vi "Dashboard Main.vi"() -> ()   [LabVIEW 2017]
uses:
  <vilib>/Utility/miscctls.llb/LVRowAndColumnTypeDef.ctl
  <vilib>/event_ctls.llb/eventvkey.ctl
  <vilib>/Rock Robotics/Network Tables/NT Read Numeric Array.vi
  <vilib>/Rock Robotics/Network Tables/NT Write Boolean.vi
  <vilib>/Rock Robotics/WPI/Dashboard/WPI_DashboardLogging Global.vi
panel:
  in  "Camera Settings Right":T1={"Frame Rate"=30, "Compression"=30, "Size"=1, "DB Camera Config"=FALSE} {"Frame Rate" scale=1.0..30.0; "Compression" scale=100.0..-1.0; "Size" items=["640x480", "320x240", "160x120"]}
  in  "Camera Name Right":string(combo)="No Camera Selection"
  out "Camera Info":cluster{"Mbps LED":bool, "Mbps":dbl, "fps":dbl} {"fps" format="%#.1g"; "Mbps" format="%#.1g"}
  in  "Camera Settings":T1={"Frame Rate"=30, "Compression"=30, "Size"=1, "DB Camera Config"=FALSE} {"Frame Rate" scale=1.0..30.0; "Compression" scale=100.0..-1.0; "Size" items=["640x480", "320x240", "160x120"]}
  in  "TCP":refnum<k5>
  in  "Rec Mode":enum32{"Stop", "Record", "Playback"}(radio)
  out "Robot IP":string
  out "Image Message":string="Timeout in Camera Communications"
  in  "Dashboard Tab":T2(tab)
  in  "Select Auto":string(combo)="Select Autonomous ..."
  out "NT Connection":bool
  out "MotorChart R":cluster{"Numeric":dbl, "Numeric":dbl}(graph)
  out "MotorChart L":cluster{"Numeric":dbl, "Numeric":dbl}(graph)
  out "MotorSliders R":cluster{"MotorSlide1":dbl, "MotorSlide2":dbl} {"MotorSlide2" scale=-1.0..1.0 scale format="%#_2e"; "MotorSlide1" scale=-1.0..1.0 scale format="%#_2e"}
  out "MotorSliders L":cluster{"MotorSlide1":dbl, "MotorSlide2":dbl} {"MotorSlide2" scale=-1.0..1.0 scale format="%#_2e"; "MotorSlide1" scale=-1.0..1.0 scale format="%#_2e"}
  out "Gyro":dbl(knob) scale=0.0..360.0
  out "JS1 Z":dbl(slide) scale=-1.0..1.0 scale format="%#_2e"
  out "JS1 Graph":cluster{"X":dbl, "Y":dbl}[](graph)
  out "JS1 Buttons":T3
  out "JS2 Z":dbl(slide) scale=-1.0..1.0 scale format="%#_2e"
  out "JS2 Graph":cluster{"X":dbl, "Y":dbl}[](graph)
  out "JS2 Buttons":T3
  out "Mode":T4(ring)=enum."Auto Disabled"
  out "Camera Image Right":T5(plugin-control)
  in  "DB/String 9":string
  in  "DB/String 8":string
  in  "DB/String 7":string
  in  "DB/String 6":string
  in  "DB/String 5":string
  in  "DB/String 4":string
  in  "DB/String 3":string
  in  "DB/String 2":string
  in  "DB/String 1":string
  in  "DB/String 0":string
  in  "DB/Slider 0":dbl(slide) scale=0.0..5.0
  in  "DB/Slider 1":dbl(slide) scale=0.0..5.0
  in  "DB/Slider 2":dbl(slide) scale=0.0..5.0
  in  "DB/Slider 3":dbl(slide) scale=0.0..5.0
  out "DB/LED 3":bool
  out "DB/LED 2":bool
  out "DB/LED 1":bool
  out "DB/LED 0":bool
  in  "DB/Button 3":bool
  in  "DB/Button 2":bool
  in  "DB/Button 1":bool
  in  "DB/Button 0":bool caption="New Name"
  out "Elev Encoder":dbl
  out "Fused Heading":dbl
  out "Right Encoder":dbl
  out "Left Encoder":dbl
  in  "Cross Line":bool
  in  "Do Nothing":bool
  in  "Cross? Button":bool
  in  "Three Cube Button":bool
  in  "Two Cube Button":bool
  in  "One Cube Button":bool
  in  "Switch Button":bool
  in  "Scale Button":bool
  in  "Right Button":bool
  in  "Center Button":bool
  in  "Left Button":bool
  out "Game Data":string
  out "AutonControl":string
  out "Reboot?":bool caption="Boolean"
  in  "Test Slider":dbl(slide) scale=0.0..100.0 scale format="%#_3g"
  in  "On/Off":bool caption="Solenoid"
  in  "Test Name":u16(ring) items=["Select the test to run..."]
  in  "Test Tree":string(tree)
  in  "Motor":cluster{"Value":dbl, "Enable":bool} {"Value" scale=-1.0..1.0 scale format="%#_3g"}
  out "Progress":T6 {"Test Progress" scale=0.0..100.0}
  in  "Rev/Fwd":cluster{"Forward":bool, "Reverse":bool}
  in  "Test Ring":u16(ring) items=["Monochrome", "Color"]
  out "Cmd Status":string
  in  "Execute Command":bool
  in  "Command Params":string[][](table)
  in  "Command Selection":i32(listbox)
  in  "CheckList":i32(listbox)
  out "Tree":string(tree)
  out "Camera Image":T5(plugin-control)
  out "Background":bool
  in  "Camera Name":string(combo)="No Camera Selection"
  # "HW"
  # "HW"
  # "Joysticks"
  # "Drive Motors"
  # "Front"
  # "Right"
  # "Left"
  # "Back"
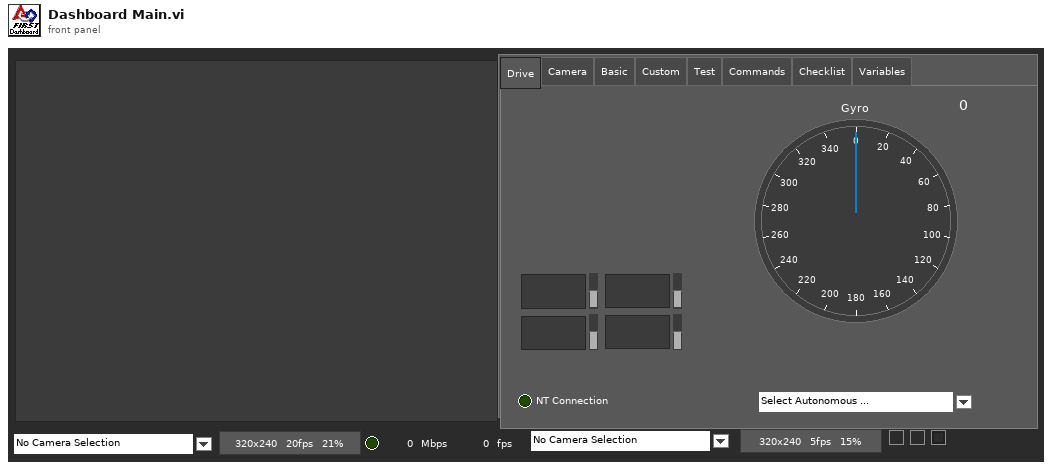
[diagram p1: front panel]
types:
  T1 = cluster{"Frame Rate":i32, "Compression":i32, "Size":u16, "DB Camera Config":bool}
  T2 = enum32{"Drive", "Camera", "Basic", "Custom", "Test", "Commands", "Checklist", "Variables"}
  T3 = cluster{bool, bool, bool, bool, bool, bool, bool, bool, bool, bool, bool, bool}
  T4 = enum8{"Tele-Op Disabled", "Tele-Op Enabled", "Auto Disabled", "Auto Enabled", "Test Disabled", "Test Enabled", "Disconnected", "No Code", "E-Stop"}
  T5 = typedef "IMAQ Image.ctl" = refnum<image>
  T6 = cluster{"Test Progress":u8, "Test Progress Text":string}
  T7 = cluster{"Save Path":path, "Interval (s)":dbl, "Keep":i32}
  T8 = typedef "Image Type" = u32
  T9 = cluster{"IDs":cluster{"RPC field ID":u16, "Unique ID":u16}, "String":string}
  T10 = cluster{"Error Strings":string, "Disable Counts":cluster{u16, u16}, "Rail Faults":cluster{u16, u16, u16}, "Robot IP":string, "DB Mode":u8, "Event Info":cluster{"Name":string, "Type":u8, "Number":u16, "Replay":u8}}
  T11 = cluster{"Storage":cluster{"Disk Free":u64, "RAM Block":u32, "RAM free":u32}, "CPU Utilization":cluster{"CPU % ISR":sgl, "CPU % Time Crit":sgl, "CPU % Timed Str":sgl, "CPU % High":sgl, "CPU % Above":sgl, "CPU % Normal":sgl, "CPU % Low":sgl}, "CAN":cluster{"% Bus Utilization":sgl, "Bus Off Cnt":u32, "TX_FIFO Full Cnt":u32, "Receive Error Cnt":u8, "Transmit Error Cnt":u8}, "HID":cluster{"HID Outputs":u32, "Rumble Low":u16, "Rumble High":u16}[]}
  T12 = cluster{"Status bits":cluster{"Test Mode":bool, "Autonomous":bool, "Enabled":bool, "Code Start":bool, "Brownout":bool, "Reserved 2":bool, "Reserved 3":bool, "E-Stop":bool}, "Code Trace":cluster{"Disabled":bool, "TeleOp":bool, "Auto":bool, "Test":bool}, "Controller Type":enum16{"unknown", "cRIO", "roboRio"}, "Code?":enum16{"unknown", "noCode", "code"}, "Battery V":dbl}
  T13 = cluster{"Control Bits":cluster{"TestMode":bool, "Autonomous":bool, "Enabled":bool, "FMS Present":bool, bool, bool, bool, "E-Stop":bool}, "Team Station ":u8, "Countdown":sgl, "Joystick Values":cluster{"Axes":dbl[], "Buttons":bool[], "POVs":i16[]}[]}
  T14 = cluster{"Axes":dbl[], "Buttons":bool[], "POVs":i16[]}[]
  T15 = cluster{"Axes":dbl[], "Buttons":bool[], "POVs":i16[]}
  T16 = cluster{"Buttons[0]":bool, "Buttons[1]":bool, "Buttons[2]":bool, "Buttons[3]":bool, "Buttons[4]":bool, "Buttons[5]":bool, "Buttons[6]":bool, "Buttons[7]":bool, "Buttons[8]":bool, "Buttons[9]":bool, "Buttons[10]":bool, "Buttons[11]":bool}
  T17 = cluster{"Camera Image":refnum<vi>, "Dashboard Tab":refnum<vi>, "Background":refnum<vi>, "Rec Mode":refnum<vi>, "Test Slider":refnum<vi>, "On/Off ":refnum<vi>, "Test Ring":refnum<vi>, "Rev/Fwd":refnum<vi>, "Test Name":refnum<vi>, "Motor":refnum<vi>, "Progress":refnum<vi>, "CheckList":refnum<vi>, "Tree":refnum<vi>, "Test Tree":refnum<vi>, "Command Params":refnum<vi>, "Command Selection":refnum<vi>, "Execute Command":refnum<vi>, "Cmd Status":refnum<vi>, "Camera Settings":refnum<vi>, "Camera Name":refnum<vi>, "Camera Info":refnum<vi>, "Camera Settings Right":refnum<vi>, "Camera Name Right":refnum<vi>, "Camera Image Right":refnum<vi>}
  T18 = cluster{"Camera Name":string, string, "Saved DB Images Info":cluster{"Save Path":path, "Interval (s)":dbl, "Keep":i32}}
  T19 = cluster{"Camera Name Right":string, string, "Saved DB Images Info":cluster{"Save Path":path, "Interval (s)":dbl, "Keep":i32}}
  T20 = cluster{"Operation":enum16{"Update", "Clear"}, "Color Box":u32}[]
  T21 = typedef "eventvkey.ctl" = enum16{"ASCII", "Enter", "Return", "Shift", "Ctrl", "Alt", "Cmd", "Opt", "Caps", "NumLock", "Clear", "Break", "Up", "Down", "Left", "Right", "Insert", "Delete", "Home", "End", "PageUp", "PageDown", "Escape", "Help", "Pause", "ScrollLock", "F1", "F2", "F3", "F4", "F5", "F6", "F7", "F8", "F9", "F10", "F11", "F12", "F13", "F14", "F15", "F16", "F17", "F18", "F19", "F20", "F21", "F22", "F23", "F24", "Play", "VolumeUp", "VolumeDown", "Mute", "Two Byte Char"}
  T22 = cluster{"Image Size":bool, "Image Type":bool, "Pixel Value":bool, "ROI Information":bool, "Zoom Factor":bool}
  T23 = cluster{"Operation":enum16{"Update", "Clear"}, "Color Box":u32}
  T24 = typedef "LVRowAndColumnTypeDef.ctl" = cluster{"Row":i32, "Column":i32}
  T25 = cluster{"Shift":bool, "Ctrl":bool, "Alt":bool, "Cmd":bool, "Opt":bool}
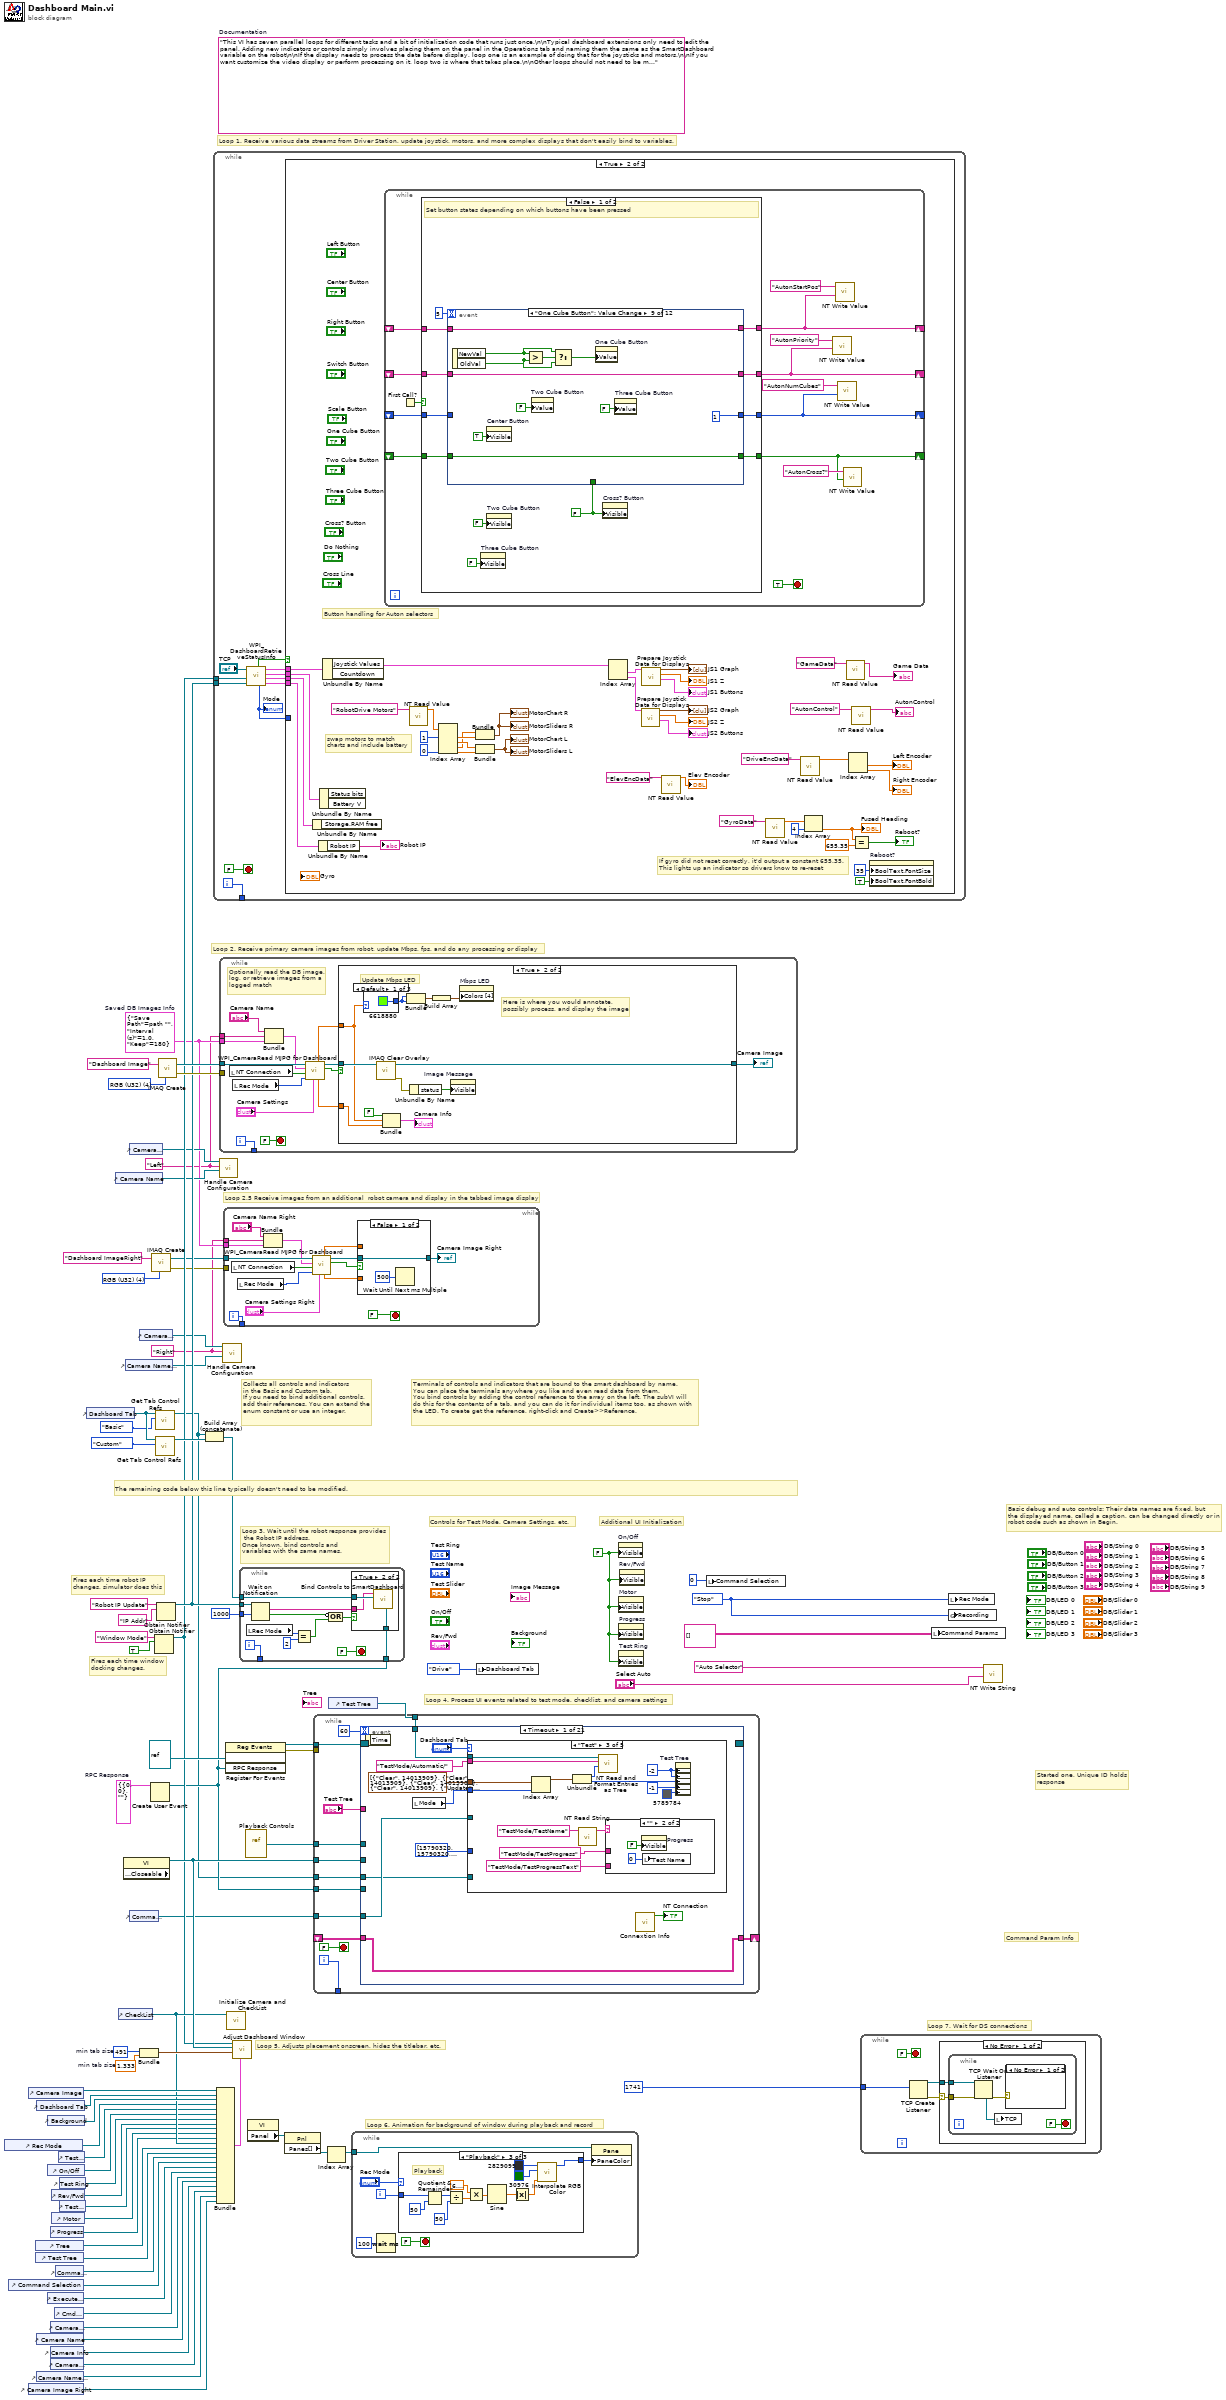
[diagram p0: block diagram]
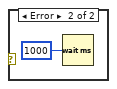
[diagram p3: hidden frame]
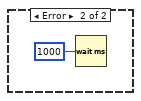
[diagram p4: hidden frame]
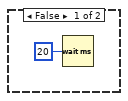
[diagram p5: hidden frame]
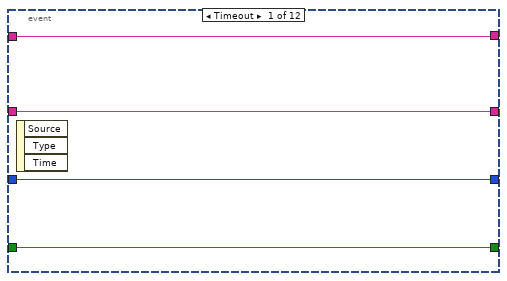
[diagram p6: hidden frame]
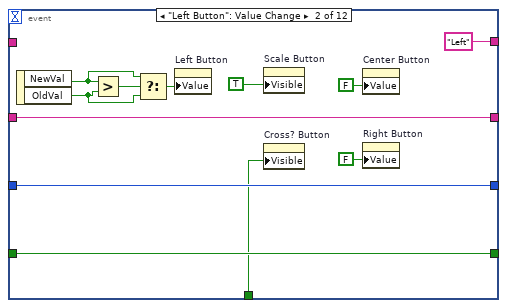
[diagram p7: hidden frame]
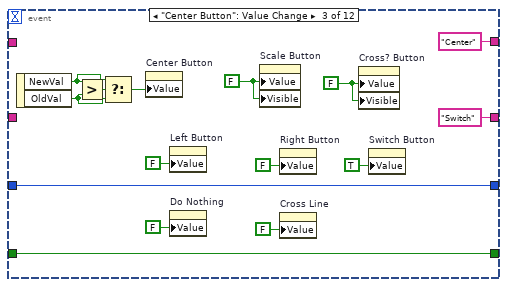
[diagram p8: hidden frame]
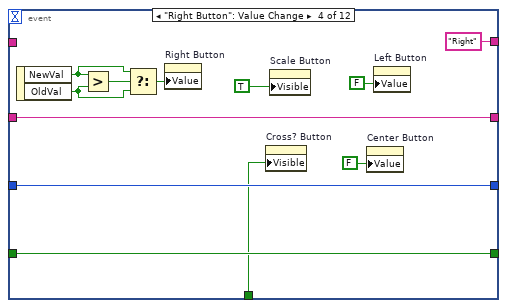
[diagram p9: hidden frame]
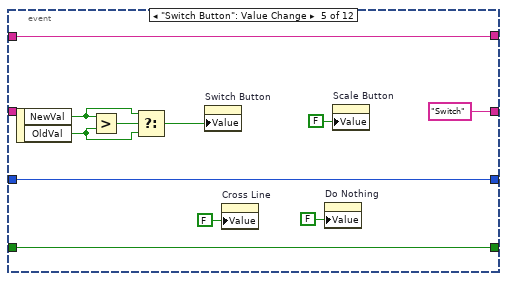
[diagram p10: hidden frame]
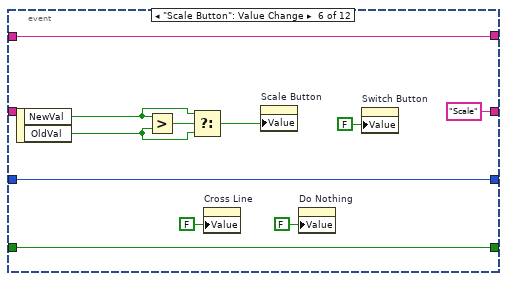
[diagram p11: hidden frame]
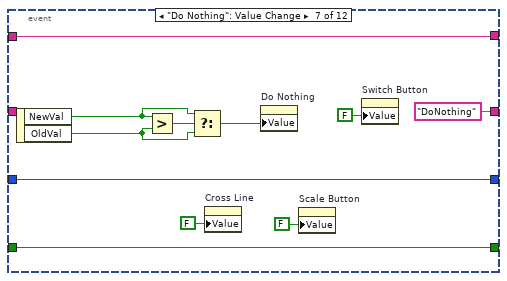
[diagram p12: hidden frame]
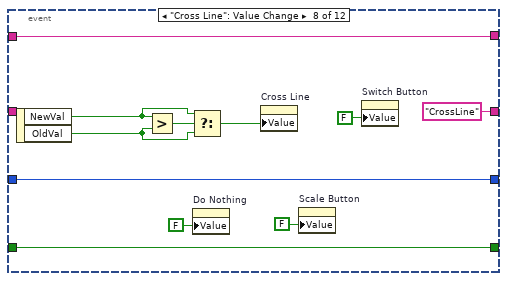
[diagram p13: hidden frame]
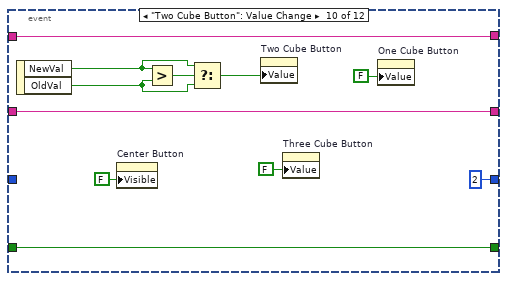
[diagram p14: hidden frame]
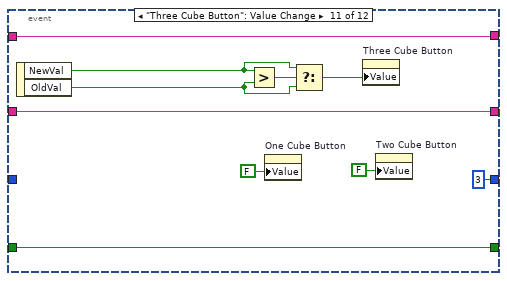
[diagram p15: hidden frame]
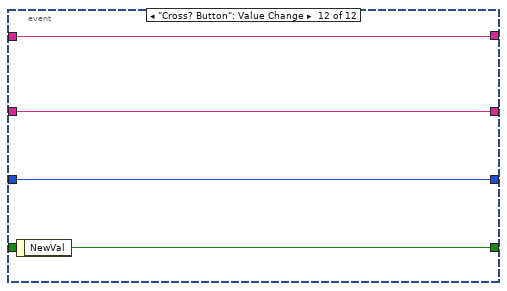
[diagram p16: hidden frame]
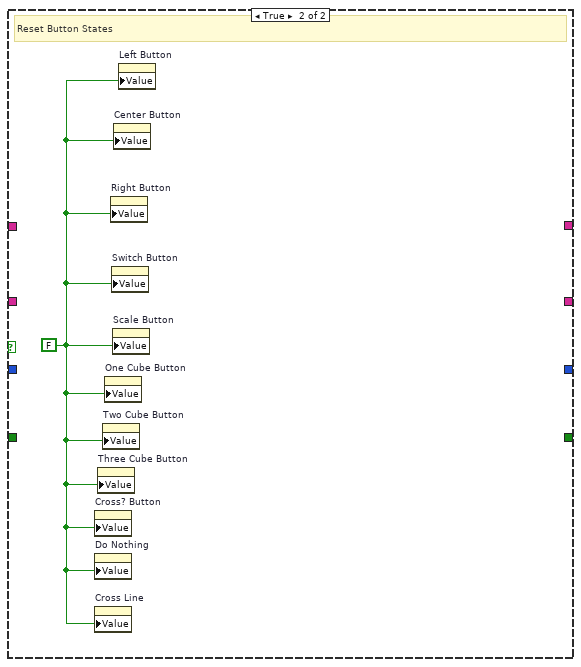
[diagram p17: hidden frame]
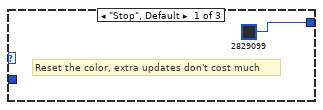
[diagram p18: hidden frame]
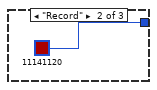
[diagram p19: hidden frame]
diagram:
  w3 = T7 {"Save Path"=path "", "Interval (s)"=1.0, "Keep"=180}  # Saved DB Images Info
  w2 = "Right"
  w1 = "Left"
  w13 = T8 4 items=["Grayscale (U8)", "Grayscale (I16)", "Grayscale (SGL)", "Complex (CSG)", "RGB (U32)", "HSL (U32)", "RGB (U64)"] ("Image Type")
  w29 = T9 {"IDs"={"RPC field ID"=0, "Unique ID"=0}, "String"=""}  # RPC Response
  w52 = 491  # min tab size
  w51 = 1.333  # min tab size
  w59 = enum32{"Stop", "Record", "Playback"}."Stop" ("Rec Mode")
  w36 = FALSE ("Visible")
  (unwired) "This VI has seven parallel loops for different tasks and a bit of initialization code that runs just once.\n\nTypical dashboard extensions only need to edit the panel. Adding new indicators or controls simply involves placing them on the panel in the Operations tab and naming them the same as the SmartDashboard variable on the robot\n\nIf the display needs to process the data before display, loop one is an example of doing that for the joysticks and motors.\n\nIf you want customize the video display or perform processing on it, loop two is where that takes place.\n\nOther loops should not need to be modified. They are pretty standard, and document the task they perform."  # Documentation
  w76 = T8 4 items=["Grayscale (U8)", "Grayscale (I16)", "Grayscale (SGL)", "Complex (CSG)", "RGB (U32)", "HSL (U32)", "RGB (U64)"] ("Image Type")
  # "Loop 2.5 Receive images from an additional  robot camera and display in the tabbed image display"
  # "Command Param Info"
  # "Started one, Unique ID holds\nresponse"
  # "Loop 7. Wait for DS connections"
  # "Basic debug and auto controls: Their data names are fixed, but\nthe displayed name, called a caption, can be changed directly or in\nrobot code such as shown in Begin."
  # "Controls for Test Mode, Camera Settings, etc."
  # "Additional UI Initialization"
  # "Loop 6. Animation for background of window during playback and record"
  # "Fires each time robot IP\nchanges, simulator does this"
  # "Fires each time window\ndocking changes."
  # "Collects all controls and indicators\nin the Basic and Custom tab.\nIf you need to bind additional controls,\nadd their references. You can extend the\nenum constant or use an integer."
  # "The remaining code below this line typically doesn't need to be modified."
  # "Loop 4. Process UI events related to test mode, checklist, and camera settings"
  # "Terminals of controls and indicators that are bound to the smart dashboard by name.\nYou can place the terminals anywhere you like and even read data from them.\nYou bind controls by adding the control reference to the array on the left. The subVI will\ndo this for the contents of a tab, and you can do it for individual items too, as shown with\nthe LED. To create get the reference, right-click and Create>>Reference."
  # "Loop 3. Wait until the robot response provides\n the Robot IP address.\nOnce known, bind controls and\nvariables with the same names."
  # "Loop 5. Adjusts placement onscreen, hides the titlebar, etc."
  # "Loop 1. Receive various data streams from Driver Station, update joystick, motors, and more complex displays that don't easily bind to variables."
  # "Loop 2. Receive primary camera images from robot, update Mbps, fps, and do any processing or display"
  n1 = control-ref of="Rec Mode"() -> (w42:refnum<vi>)
  n2 = control-ref of="Command Selection"() -> (w28:refnum<vi>)
  n3 = control-ref of="Camera Image Right"() -> (w6:refnum<vi>)
  n4 = control-ref of="Camera Image"() -> (w54:refnum<vi>)
  n5 = control-ref of="Tree"() -> (w46:refnum<vi>)
  n6 = control-ref of="Test Tree"() -> (w45:refnum<vi>)
  n7 = control-ref of="Dashboard Tab"() -> (w53:refnum<vi>)
  n8 = control-ref of="Camera Name"() -> (w19:refnum<vi>)
  n9 = control-ref of="Camera Name Right"() -> (w7:refnum<vi>)
  n10 = control-ref of="Execute Command"() -> (w30:refnum<vi>)
  n11 = control-ref of="Background"() -> (w49:refnum<vi>)
  n12 = control-ref of="On/Off"() -> (w40:refnum<vi>)
  n13 = control-ref of="Progress"() -> (w37:refnum<vi>)
  n14 = control-ref of="Camera Settings"() -> (w20:refnum<vi>)
  n15 = control-ref of="Camera Info"() -> (w18:refnum<vi>)
  n16 = control-ref of="Camera Settings Right"() -> (w8:refnum<vi>)
  n17 = control-ref of="Rev/Fwd"() -> (w38:refnum<vi>)
  n18 = control-ref of="Motor"() -> (w43:refnum<vi>)
  n19 = control-ref of="Cmd Status"() -> (w24:refnum<vi>)
  n20 = control-ref of="Command Params"() -> (w31:refnum<vi>)
  n21 = control-ref of="Test Slider"() -> (w41:refnum<vi>)
  n22 = control-ref of="Test Ring"() -> (w39:refnum<vi>)
  n23 = control-ref of="Test Name"() -> (w44:refnum<vi>)
  n24 = control-ref of="Dashboard Tab"() -> (w57:refnum<vi>)
  n25 = control-ref of="Camera Name"() -> (w21:refnum<vi>)
  n26 = control-ref of="CheckList"() -> (w47:refnum<vi>)
  n27 = property class="VI" props=["Front Panel.Closeable"]() -> (reference out=w58:refnum<vi>)  [unwired: 2 in, 2 out]
  n28 = control-ref of="Camera Name Right"() -> (w9:refnum<vi>)
  n29 = control-ref of="Camera Settings"() -> (w22:refnum<vi>)
  n30 = control-ref of="Command Params"() -> (w23:refnum<vi>)
  n31 = control-ref of="Camera Settings Right"() -> (w10:refnum<vi>)
  n32 = Bundle("min tab size"=w52, "min tab size"=w51) -> (w50:cluster{"min tab size":i32, "min tab size":dbl})  [unwired: 1 in]
  n33 = Create User Event(user event datatype=w29) -> (user event=w25:refnum<user-event>)  [unwired: 1 in, 1 out]
  n34 = call "IMAQ Create"("Image Name"="Dashboard ImageRight", "Image Type"=w13) -> ("New Image"=w12:T5, "error out"=w11:errorcluster)  [unwired: 2 in, 1 out]
  n35 = Obtain Notifier(name (unnamed)="Window Mode", notification data type=TRUE) -> (notifier out=w34:refnum<notifier>)  [unwired: 2 in, 2 out]
  n36 = call <vilib>:"Get Tab Control Refs.vi"("Page Index"=T2."Basic" ("Dashboard Tab"), "TabControl in"=w57) -> ("ControlsOnPage"=w17:refnum<vi>[])  [unwired: 9 in]
  n37 = call <vilib>:"Get Tab Control Refs.vi"("Page Index"=T2."Custom" ("Dashboard Tab"), "TabControl in"=w57) -> ("ControlsOnPage"=w56:refnum<vi>[])  [unwired: 9 in]
  n38 = Obtain Notifier(name (unnamed)="Robot IP Update", notification data type="IP Addr" ("name (unnamed)")) -> (notifier out=w35:refnum<notifier>)  [unwired: 2 in, 2 out]
  n39 = call "IMAQ Create"("Image Name"="Dashboard Image", "Image Type"=w76) -> ("New Image"=w74:T5, "error out"=w73:errorcluster)  [unwired: 2 in, 1 out]
  n40 = Build Array (concatenate)(w17, w56) -> (w55:refnum<vi>[])
  n41 = while {
    tunnel: [w86] -> _
    tunnel: w35 -> [w80]
    tunnel: w34 -> [w77]
    i -> [w86]
    stop <- FALSE stop-if-true
    n42 = call <vilib>:"WPI_DashboardRetrieveStatusInfo.vi"("Binding Refnum"=w80, "Window Mode Notifier"=w77, "TCP Cnx"="TCP") -> ("Power and Errors"=w81:T10, "Robot Metrics"=w84:T11, "Status Info"=w85:T12, "Control Info"=w82:T13, "Robot Mode"=w79:T4, "Process?"=w83:bool)  [unwired: 3 in]
    "Mode" <- w79
    n43 = case shown="True" w83 {
      tunnel: w85 -> [_ w130]
      tunnel: w84 -> [_ w129]
      tunnel: w82 -> [_ w128]
      tunnel: w81 -> [_ w127]
      tunnel: w79 -> [_ _]
      frame False {
        n44 = Wait (ms)(milliseconds to wait=u32 20) -> ()  [unwired: 1 out]
      }
      frame True {
        # "Button handling for Auton selectors"
        # "If gyro did not reset correctly, it'd output a constant 655.35.  This lights up an indicator so drivers know to re-reset"
        # "swap motors to match\ncharts and include battery"
        n45 = Unbundle By Name(w129) -> ()  [unwired: 1 out]
        n46 = Unbundle By Name(w127) -> ("Robot IP"=→"Robot IP":string)
        n47 = Unbundle By Name(w130) -> ()  [unwired: 2 out]
        n48 = Unbundle By Name(w128) -> ("Joystick Values"=w118:T14)  [unwired: 1 out]
        n49 = while {
          shift-right: [w138] -> _
          shift-left: _ -> [w144]
          shift-right: [w134] -> _
          shift-left: _ -> [w143]
          shift-right: [w136] -> _
          shift-left: _ -> [w142]
          shift-right: [w133] -> _
          shift-left: _ -> [w132]
          stop <- TRUE stop-if-true
          n50 = First Call?() -> (First Call?: T/F=w131:bool)
          n51 = case shown="False" w131 {
            tunnel: [w156 _] -> w138
            tunnel: [w155 _] -> w134
            tunnel: w144 -> [w154 _]
            tunnel: w143 -> [w153 _]
            tunnel: w142 -> [w152 _]
            tunnel: [w151 _] -> w136
            tunnel: [w150 _] -> w133
            tunnel: w132 -> [w149 _]
            frame False {
              w146 = FALSE ("Center Button")
              # "Set button states depending on which buttons have been pressed"
              n52 = event shown="[8] \"One Cube Button\": Value Change" {
                selector: _ -> [_ _ _ _ _ _ _ _ _ _ _ _]
                dyn-events: _ -> [_ _ _ _ _ _ _ _ _ _ _ _]
                timeout: 5 -> [_ _ _ _ _ _ _ _ _ _ _ _]
                tunnel: [w160 "Left" "Center" "Right" w204 w215 w226 w237 w248 w258 w269 w276] -> w156
                tunnel: [w159 w164 "Switch" w191 "Switch" "Scale" "DoNothing" "CrossLine" w247 w259 w268 w277] -> w155
                tunnel: w154 -> [w160 _ _ _ w204 w215 w226 w237 w248 w258 w269 w276]
                tunnel: w153 -> [w159 w164 _ w191 _ _ _ _ w247 w259 w268 w277]
                tunnel: w152 -> [w158 w163 w176 w190 w203 w214 w225 w236 _ _ _ w278]
                tunnel: [w158 w163 w176 w190 w203 w214 w225 w236 1 2 3 w278] -> w151
                tunnel: [w157 w162 w175 w189 w200 w211 w222 w233 w245 w256 w266 w279] -> w150
                tunnel: w149 -> [w157 w162 w175 w189 w200 w211 w222 w233 w245 w256 w266 _]
                tunnel: w146 -> [_ w161 _ w188 _ _ _ _ _ _ _ _]
                event Timeout {
                  n53 = event-data() -> ()  [unwired: 1 in, 3 out]
                }
                event "Left Button": Value Change {
                  n54 = event-data() -> ("NewVal"=w169:bool, "OldVal"=w168:bool)  [unwired: 1 in]
                  n55 = Greater?(x=w169, y=w168) -> (0:w170:bool)
                  n56 = Select(t=w169, s=w170, f=w168) -> (s? t:f=w167:bool)
                  n57 = property on="Left Button" class="Bool (strict)"("Value"=w167) -> ()  [unwired: 2 in, 2 out]
                  n58 = property on="Scale Button" class="Bool (strict)"("Visible"=TRUE ("Right Button")) -> ()  [unwired: 2 in, 2 out]
                  n59 = property on="Cross? Button" class="Bool (strict)"("Visible"=w161) -> ()  [unwired: 2 in, 2 out]
                  n60 = property on="Center Button" class="Bool (strict)"("Value"=FALSE ("Center Button")) -> ()  [unwired: 2 in, 2 out]
                  n61 = property on="Right Button" class="Bool (strict)"("Value"=FALSE ("Right Button")) -> ()  [unwired: 2 in, 2 out]
                }
                event "Center Button": Value Change {
                  w180 = FALSE ("Right Button")
                  w179 = FALSE ("Right Button")
                  n62 = event-data() -> ("NewVal"=w182:bool, "OldVal"=w183:bool)  [unwired: 1 in]
                  n63 = Greater?(x=w182, y=w183) -> (0:w185:bool)
                  n64 = Select(t=w182, s=w185, f=w183) -> (s? t:f=w184:bool)
                  n65 = property on="Center Button" class="Bool (strict)"("Value"=w184) -> ()  [unwired: 2 in, 2 out]
                  n66 = property on="Left Button" class="Bool (strict)"("Value"=FALSE ("Center Button")) -> ()  [unwired: 2 in, 2 out]
                  n67 = property on="Do Nothing" class="Bool (strict)"("Value"=FALSE ("Center Button")) -> ()  [unwired: 2 in, 2 out]
                  n68 = property on="Scale Button" class="Bool (strict)"("Value"=w179, "Visible"=w179) -> ()  [unwired: 2 in, 2 out]
                  n69 = property on="Right Button" class="Bool (strict)"("Value"=FALSE ("Right Button")) -> ()  [unwired: 2 in, 2 out]
                  n70 = property on="Cross Line" class="Bool (strict)"("Value"=FALSE ("Right Button")) -> ()  [unwired: 2 in, 2 out]
                  n71 = property on="Cross? Button" class="Bool (strict)"("Value"=w180, "Visible"=w180) -> ()  [unwired: 2 in, 2 out]
                  n72 = property on="Switch Button" class="Bool (strict)"("Value"=TRUE ("Right Button")) -> ()  [unwired: 2 in, 2 out]
                }
                event "Right Button": Value Change {
                  n73 = event-data() -> ("NewVal"=w194:bool, "OldVal"=w195:bool)  [unwired: 1 in]
                  n74 = Greater?(x=w194, y=w195) -> (0:w197:bool)
                  n75 = Select(t=w194, s=w197, f=w195) -> (s? t:f=w196:bool)
                  n76 = property on="Right Button" class="Bool (strict)"("Value"=w196) -> ()  [unwired: 2 in, 2 out]
                  n77 = property on="Cross? Button" class="Bool (strict)"("Visible"=w188) -> ()  [unwired: 2 in, 2 out]
                  n78 = property on="Scale Button" class="Bool (strict)"("Visible"=TRUE ("Right Button")) -> ()  [unwired: 2 in, 2 out]
                  n79 = property on="Center Button" class="Bool (strict)"("Value"=FALSE ("Right Button")) -> ()  [unwired: 2 in, 2 out]
                  n80 = property on="Left Button" class="Bool (strict)"("Value"=FALSE ("Center Button")) -> ()  [unwired: 2 in, 2 out]
                }
                event "Switch Button": Value Change {
                  n81 = event-data() -> ("NewVal"=w206:bool, "OldVal"=w207:bool)  [unwired: 1 in]
                  n82 = Greater?(x=w206, y=w207) -> (0:w209:bool)
                  n83 = Select(t=w206, s=w209, f=w207) -> (s? t:f=w208:bool)
                  n84 = property on="Switch Button" class="Bool (strict)"("Value"=w208) -> ()  [unwired: 2 in, 2 out]
                  n85 = property on="Cross Line" class="Bool (strict)"("Value"=FALSE ("Center Button")) -> ()  [unwired: 2 in, 2 out]
                  n86 = property on="Do Nothing" class="Bool (strict)"("Value"=FALSE ("Center Button")) -> ()  [unwired: 2 in, 2 out]
                  n87 = property on="Scale Button" class="Bool (strict)"("Value"=FALSE ("Center Button")) -> ()  [unwired: 2 in, 2 out]
                }
                event "Scale Button": Value Change {
                  n88 = event-data() -> ("NewVal"=w217:bool, "OldVal"=w218:bool)  [unwired: 1 in]
                  n89 = Greater?(x=w217, y=w218) -> (0:w220:bool)
                  n90 = Select(t=w217, s=w220, f=w218) -> (s? t:f=w219:bool)
                  n91 = property on="Cross Line" class="Bool (strict)"("Value"=FALSE ("Center Button")) -> ()  [unwired: 2 in, 2 out]
                  n92 = property on="Scale Button" class="Bool (strict)"("Value"=w219) -> ()  [unwired: 2 in, 2 out]
                  n93 = property on="Do Nothing" class="Bool (strict)"("Value"=FALSE ("Center Button")) -> ()  [unwired: 2 in, 2 out]
                  n94 = property on="Switch Button" class="Bool (strict)"("Value"=FALSE ("Center Button")) -> ()  [unwired: 2 in, 2 out]
                }
                event "Do Nothing": Value Change {
                  n95 = event-data() -> ("NewVal"=w228:bool, "OldVal"=w229:bool)  [unwired: 1 in]
                  n96 = Greater?(x=w228, y=w229) -> (0:w231:bool)
                  n97 = Select(t=w228, s=w231, f=w229) -> (s? t:f=w230:bool)
                  n98 = property on="Cross Line" class="Bool (strict)"("Value"=FALSE ("Center Button")) -> ()  [unwired: 2 in, 2 out]
                  n99 = property on="Do Nothing" class="Bool (strict)"("Value"=w230) -> ()  [unwired: 2 in, 2 out]
                  n100 = property on="Scale Button" class="Bool (strict)"("Value"=FALSE ("Center Button")) -> ()  [unwired: 2 in, 2 out]
                  n101 = property on="Switch Button" class="Bool (strict)"("Value"=FALSE ("Center Button")) -> ()  [unwired: 2 in, 2 out]
                }
                event "Cross Line": Value Change {
                  n102 = event-data() -> ("NewVal"=w239:bool, "OldVal"=w240:bool)  [unwired: 1 in]
                  n103 = Greater?(x=w239, y=w240) -> (0:w242:bool)
                  n104 = Select(t=w239, s=w242, f=w240) -> (s? t:f=w241:bool)
                  n105 = property on="Do Nothing" class="Bool (strict)"("Value"=FALSE ("Center Button")) -> ()  [unwired: 2 in, 2 out]
                  n106 = property on="Cross Line" class="Bool (strict)"("Value"=w241) -> ()  [unwired: 2 in, 2 out]
                  n107 = property on="Scale Button" class="Bool (strict)"("Value"=FALSE ("Center Button")) -> ()  [unwired: 2 in, 2 out]
                  n108 = property on="Switch Button" class="Bool (strict)"("Value"=FALSE ("Center Button")) -> ()  [unwired: 2 in, 2 out]
                }
                event "One Cube Button": Value Change {
                  n109 = event-data() -> ("NewVal"=w250:bool, "OldVal"=w251:bool)  [unwired: 1 in]
                  n110 = property on="Center Button" class="Bool (strict)"("Visible"=TRUE ("Center Button")) -> ()  [unwired: 2 in, 2 out]
                  n111 = Greater?(x=w250, y=w251) -> (0:w253:bool)
                  n112 = property on="Two Cube Button" class="Bool (strict)"("Value"=FALSE ("Center Button")) -> ()  [unwired: 2 in, 2 out]
                  n113 = Select(t=w250, s=w253, f=w251) -> (s? t:f=w252:bool)
                  n114 = property on="One Cube Button" class="Bool (strict)"("Value"=w252) -> ()  [unwired: 2 in, 2 out]
                  n115 = property on="Three Cube Button" class="Bool (strict)"("Value"=FALSE ("Center Button")) -> ()  [unwired: 2 in, 2 out]
                }
                event "Two Cube Button": Value Change {
                  n116 = event-data() -> ("NewVal"=w261:bool, "OldVal"=w262:bool)  [unwired: 1 in]
                  n117 = property on="Center Button" class="Bool (strict)"("Visible"=FALSE ("Center Button")) -> ()  [unwired: 2 in, 2 out]
                  n118 = Greater?(x=w261, y=w262) -> (0:w264:bool)
                  n119 = Select(t=w261, s=w264, f=w262) -> (s? t:f=w263:bool)
                  n120 = property on="Two Cube Button" class="Bool (strict)"("Value"=w263) -> ()  [unwired: 2 in, 2 out]
                  n121 = property on="Three Cube Button" class="Bool (strict)"("Value"=FALSE ("Center Button")) -> ()  [unwired: 2 in, 2 out]
                  n122 = property on="One Cube Button" class="Bool (strict)"("Value"=FALSE ("Center Button")) -> ()  [unwired: 2 in, 2 out]
                }
                event "Three Cube Button": Value Change {
                  n123 = event-data() -> ("NewVal"=w271:bool, "OldVal"=w272:bool)  [unwired: 1 in]
                  n124 = Greater?(x=w271, y=w272) -> (0:w274:bool)
                  n125 = property on="One Cube Button" class="Bool (strict)"("Value"=FALSE ("Center Button")) -> ()  [unwired: 2 in, 2 out]
                  n126 = Select(t=w271, s=w274, f=w272) -> (s? t:f=w273:bool)
                  n127 = property on="Three Cube Button" class="Bool (strict)"("Value"=w273) -> ()  [unwired: 2 in, 2 out]
                  n128 = property on="Two Cube Button" class="Bool (strict)"("Value"=FALSE ("Center Button")) -> ()  [unwired: 2 in, 2 out]
                }
                event "Cross? Button": Value Change {
                  n129 = event-data() -> ("NewVal"=w279:bool)  [unwired: 1 in]
                }
              }
              n130 = property on="Three Cube Button" class="Bool (strict)"("Visible"=FALSE ("Center Button")) -> ()  [unwired: 2 in, 2 out]
              n131 = property on="Two Cube Button" class="Bool (strict)"("Visible"=FALSE ("Center Button")) -> ()  [unwired: 2 in, 2 out]
              n132 = property on="Cross? Button" class="Bool (strict)"("Visible"=w146) -> ()  [unwired: 2 in, 2 out]
            }
            frame True {
              w280 = FALSE
              # "Reset Button States"
              n133 = property on="Cross? Button" class="Bool (strict)"("Value"=w280) -> ()  [unwired: 2 in, 2 out]
              n134 = property on="Do Nothing" class="Bool (strict)"("Value"=w280) -> ()  [unwired: 2 in, 2 out]
              n135 = property on="Cross Line" class="Bool (strict)"("Value"=w280) -> ()  [unwired: 2 in, 2 out]
              n136 = property on="Three Cube Button" class="Bool (strict)"("Value"=w280) -> ()  [unwired: 2 in, 2 out]
              n137 = property on="Two Cube Button" class="Bool (strict)"("Value"=w280) -> ()  [unwired: 2 in, 2 out]
              n138 = property on="One Cube Button" class="Bool (strict)"("Value"=w280) -> ()  [unwired: 2 in, 2 out]
              n139 = property on="Right Button" class="Bool (strict)"("Value"=w280) -> ()  [unwired: 2 in, 2 out]
              n140 = property on="Switch Button" class="Bool (strict)"("Value"=w280) -> ()  [unwired: 2 in, 2 out]
              n141 = property on="Scale Button" class="Bool (strict)"("Value"=w280) -> ()  [unwired: 2 in, 2 out]
              n142 = property on="Center Button" class="Bool (strict)"("Value"=w280) -> ()  [unwired: 2 in, 2 out]
              n143 = property on="Left Button" class="Bool (strict)"("Value"=w280) -> ()  [unwired: 2 in, 2 out]
            }
          }
          n144 = call-poly <vilib>:"NT Write Value.vi"("String"=w134, "Name"="AutonPriority") -> ()  [unwired: 9 in, 1 out]
          n145 = call-poly <vilib>:"NT Write Value.vi"("String"=w138, "Name"="AutonStartPos") -> ()  [unwired: 9 in, 1 out]
          n146 = call-poly <vilib>:"NT Write Value.vi"("Numeric"=w136, "Name"="AutonNumCubes") -> ()  [unwired: 9 in, 1 out]
          n147 = call-poly <vilib>:"NT Write Value.vi"("Boolean"=w133, "Name"="AutonCross?") -> ()  [unwired: 9 in, 1 out]
        }
        n148 = call-poly <vilib>:"NT Read Value.vi"("Name"="RobotDrive Motors") -> ("Numeric Array"=w108:dbl[])  [unwired: 9 in, 1 out]
        n149 = Index Array(array=w108, index #1=1, index #4=0) -> (element #1=w122:dbl, element #2=w123:dbl, element #3=w121:dbl, element #4=w126:dbl)  [unwired: 2 in]
        n150 = Bundle("Numeric"=w121, "Numeric"=w122) -> (→"MotorChart R" →"MotorSliders R":cluster{"Numeric":dbl, "Numeric":dbl})  [unwired: 1 in]
        n151 = Bundle("Numeric"=w123, "Numeric"=w126) -> (→"MotorChart L" →"MotorSliders L":cluster{"Numeric":dbl, "Numeric":dbl})  [unwired: 1 in]
        n152 = Index Array(array=w118) -> (element #1=w117:T15, element #2=w113:T15)  [unwired: 2 in]
        n153 = call "Prepare Joystick Data for Displays.vi"("Joystick Values"=w113) -> ("Buttons"=→"JS2 Buttons":T16, "Z Axis"=→"JS2 Z":dbl, "Cartesian Data"=→"JS2 Graph":cluster{"X axis":dbl, "X axis":dbl}[])  [unwired: 8 in]
        n154 = call "Prepare Joystick Data for Displays.vi"("Joystick Values"=w117) -> ("Buttons"=→"JS1 Buttons":T16, "Z Axis"=→"JS1 Z":dbl, "Cartesian Data"=→"JS1 Graph":cluster{"X axis":dbl, "X axis":dbl}[])  [unwired: 8 in]
        n155 = call-poly <vilib>:"NT Read Value.vi"("Name"="ElevEncData") -> ("Numeric"=→"Elev Encoder":dbl)  [unwired: 9 in, 1 out]
        n156 = call-poly <vilib>:"NT Read Value.vi"("Name"="GyroData") -> ("Numeric Array"=w100:dbl[])  [unwired: 9 in, 1 out]
        n157 = call-poly <vilib>:"NT Read Value.vi"("Name"="DriveEncData") -> ("Numeric Array"=w98:dbl[])  [unwired: 9 in, 1 out]
        n158 = Index Array(array=w100, index=4) -> (element=w93:dbl)
        "Fused Heading" <- w93
        n159 = call-poly <vilib>:"NT Read Value.vi"("Name"="GameData") -> ("String"=→"Game Data":string)  [unwired: 9 in, 1 out]
        n160 = Index Array(array=w98) -> (element #1=→"Left Encoder":dbl, element #2=→"Right Encoder":dbl)  [unwired: 2 in]
        n161 = call-poly <vilib>:"NT Read Value.vi"("Name"="AutonControl") -> ("String"=→"AutonControl":string)  [unwired: 9 in, 1 out]
        n162 = Equal?(x=w93, y=655.35) -> (x = y?=→"Reboot?":bool)
        n163 = property on="Reboot?" class="Bool (strict)"("BoolText.FontSize"=u32 35 ("Boolean Text.Font:Size"), "BoolText.FontBold"=TRUE ("Boolean Text.Font:Bold")) -> ()  [unwired: 2 in, 2 out]
      }
    }
  }
  n164 = Bundle("Camera Image"=w54, "Dashboard Tab"=w53, "Background"=w49, "Rec Mode"=w42, "Test Slider"=w41, "On/Off"=w40, "Test Ring"=w39, "Rev/Fwd"=w38, "Test Name"=w44, "Motor"=w43, "Progress"=w37, "CheckList"=w47, "Tree"=w46, "Test Tree"=w45, "Command Params"=w31, "Command Selection"=w28, "Execute Command"=w30, "Cmd Status"=w24, "Camera Settings"=w20, "Camera Name"=w19, "Camera Info"=w18, "Camera Settings Right"=w8, "Camera Name Right"=w7, "Camera Image Right"=w6) -> (w48:T17)  [unwired: 1 in]
  n165 = call "Handle Camera Configuration.vi"("CameraNameRef"=w21, "Display Name"=w1, "ClusterRef"=w22) -> ()  [unwired: 9 in]
  n166 = while {
    tunnel: w74 -> [w293]
    tunnel: w73 -> [_]
    tunnel: [w294] -> _
    tunnel: w3 -> [w284]
    tunnel: w1 -> [w281]
    i -> [w294]
    stop <- FALSE stop-if-true
    # "Optionally read the DB image,\nlog, or retrieve images from a\nlogged match"
    n167 = local read "NT Connection"() -> (w285:bool)
    n168 = local read "Rec Mode"() -> (w289:enum32{"Stop", "Record", "Playback"})
    n169 = Bundle("Camera Name"="Camera Name", w281, "Saved DB Images Info"=w284) -> (w283:T18)  [unwired: 1 in]
    n170 = call <vilib>:"WPI_CameraRead MJPG for Dashboard.vi"("Camera Settings"="Camera Settings", "Rec Mode"=w289, "NT Connection"=w285, "Capture Info"=w283, "Refnum in"=w293) -> ("Active"=w291:bool, "Refnum out"=w292:T5, "FPS"=w290:dbl, "Bandwidth (Mbps)"=w288:dbl)  [unwired: 3 in]
    n171 = case shown="True" w291 {
      tunnel: w292 -> [w296 w307]
      tunnel: w288 -> [_ w304]
      tunnel: w290 -> [_ w305]
      tunnel: [w296 w301] -> w286
      frame False {
        w298 = u32 1985280 ("Color Box")
        # "Sleep for 500ms"
        n172 = Bundle("Color Box"=w298, "Color Box"=w298) -> (w299:cluster{"Color Box":u32, "Color Box":u32})  [unwired: 1 out]
        n173 = Build Array(w299) -> (w297:cluster{"Color Box":u32, "Color Box":u32}[])
        n174 = property on="Mbps LED" class="Bool (strict)"("Colors [4]"=w297) -> ()  [unwired: 2 in, 2 out]
        n175 = Wait Until Next ms Multiple(millisecond multiple=u32 500) -> ()  [unwired: 1 out]
      }
      frame True {
        # "Here is where you would annotate,\npossibly process, and display the image"
        # "Update Mbps LED"
        n176 = case shown="Default" w304 {
          tunnel: [u32 6618880 ("Color Box") u32 16776722 ("Color Box") u32 16716800 ("Color Box")] -> w308
          frame Default {
          }
          frame 4, 5 {
          }
          frame 6.. {
          }
        }
        n177 = call "IMAQ Clear Overlay"("Image"=w307) -> ("error out"=w310:errorcluster, "Image Out"=w301:T5)  [unwired: 2 in, 7 out]
        n178 = Bundle(FALSE, "Bandwidth (Mbps)"=w304, "FPS"=w305) -> (→"Camera Info":cluster{bool, "Bandwidth (Mbps)":dbl, "FPS":dbl})  [unwired: 1 in]
        n179 = Bundle("Color Box"=w308, "Color Box"=w308) -> (w309:cluster{"Color Box":u32, "Color Box":u32})  [unwired: 1 out]
        n180 = Unbundle By Name(w310) -> ("status"=w311:bool)
        n181 = Build Array(w309) -> (w306:cluster{"Color Box":u32, "Color Box":u32}[])
        n182 = property on="Image Message" class="Str"("Visible"=w311) -> ()  [unwired: 2 in, 2 out]
        n183 = property on="Mbps LED" class="Bool (strict)"("Colors [4]"=w306) -> ()  [unwired: 2 in, 2 out]
      }
    }
    "Camera Image" <- w286
  }
  n184 = call "Handle Camera Configuration.vi"("CameraNameRef"=w9, "Display Name"=w2, "ClusterRef"=w10) -> ()  [unwired: 9 in]
  n185 = while {
    tunnel: w12 -> [w329]
    tunnel: w11 -> [_]
    tunnel: [w324] -> _
    tunnel: w3 -> [w318]
    tunnel: w2 -> [w315]
    i -> [w324]
    stop <- FALSE stop-if-true
    n186 = local read "NT Connection"() -> (w319:bool)
    n187 = local read "Rec Mode"() -> (w328:enum32{"Stop", "Record", "Playback"})
    n188 = Bundle("Camera Name Right"="Camera Name Right", w315, "Saved DB Images Info"=w318) -> (w317:T19)  [unwired: 1 in]
    n189 = call <vilib>:"WPI_CameraRead MJPG for Dashboard.vi"("Camera Settings"="Camera Settings Right", "Rec Mode"=w328, "NT Connection"=w319, "Capture Info"=w317, "Refnum in"=w329) -> ("Active"=w323:bool, "Refnum out"=w326:T5, "FPS"=w321:dbl, "Bandwidth (Mbps)"=w322:dbl)  [unwired: 3 in]
    n190 = case shown="False" w323 {
      tunnel: w326 -> [w330 w332]
      tunnel: w322 -> [_ _]
      tunnel: w321 -> [_ _]
      tunnel: [w330 w332] -> w320
      frame False {
        n191 = Wait Until Next ms Multiple(millisecond multiple=u32 500) -> ()  [unwired: 1 out]
      }
      frame True {
      }
    }
    "Camera Image Right" <- w320
  }
  n192 = register-events(refnum<vi> refnum, w25) -> (reference out=w63:refnum<event-registration>, error out=w62:errorcluster)  [unwired: 2 in]
  n193 = call "Initialize Camera and CheckList.vi"("ListBox in"=w47) -> ()  [unwired: 11 in]
  n194 = call "Adjust Dashboard Window.vi"("Sizing Refnums"=w48, "Size Constraints"=w50, "VI"=w58, "WIn Mode"=w34) -> ()  [unwired: 8 in]
  n195 = while {
    tunnel: w55 -> [w344]
    tunnel: w35 -> [w342]
    tunnel: [w340] -> _
    tunnel: u32 1000 ("milliseconds to wait") -> [w339]
    tunnel: w25 -> [w333]
    i -> [w340]
    stop <- FALSE stop-if-true
    n196 = local read "Rec Mode"() -> (w335:enum32{"Stop", "Record", "Playback"})
    n197 = Wait on Notification(notifier=w342, timeout in ms (-1)=w339) -> (notification=w341:string, timed out?=w337:bool)  [unwired: 2 in, 2 out]
    n198 = Equal?(x=w335, y=u16 2 ("Rec Mode")) -> (x = y?=w336:bool)
    n199 = Compound Arithmetic op=OR(invert w337, w336) -> (w338:bool)
    n200 = case shown="True" w338 {
      tunnel: w344 -> [_ w347]
      tunnel: w341 -> [_ w346]
      tunnel: w333 -> [_ w345]
      frame False {
      }
      frame True {
        n201 = call <vilib>:"Bind Controls to SmartDashboard.vi"("RPC ref"=w345, "Bound Control Refs"=w347, "Server IP Address"=w346) -> ()  [unwired: 9 in]
      }
    }
  }
  n202 = vi-ref "Playback Controls.vi"() -> (w64:refnum<vi>)
  n203 = property class="VI"() -> ("Panel"=w66:refnum<vi>)  [unwired: 2 in, 2 out]
  n204 = property class="Pnl"(reference=w66) -> ("Panes[]"=w67:refnum<vi>[])  [unwired: 1 in, 2 out]
  n205 = Index Array(array=w67) -> (element=w65:refnum<vi>)  [unwired: 1 in]
  n206 = control-ref of="Test Tree"() -> (w68:refnum<vi>)
  n207 = while {
    tunnel: [w357] -> _
    tunnel: w68 -> [w356]
    tunnel: w64 -> [w355]
    tunnel: w63 -> [w354]
    tunnel: w62 -> [_]
    tunnel: w58 -> [w353]
    tunnel: w25 -> [w352]
    tunnel: w23 -> [w351]
    shift-right: [w350] -> _
    shift-left: _ -> [w349]
    tunnel: w17 -> [w348]
    i -> [w357]
    stop <- FALSE stop-if-true
    n208 = event shown="[0] Timeout" {
      selector: w354 -> [_ _ _ _ _ _ _ _ _ _ _ _ _ _ _ _ _ _ _ _ _]
      dyn-events: [_ _ _ _ _ _ _ _ _ _ _ _ _ _ _ _ w617 _ _ _ _] -> _
      timeout: u32 60 ("milliseconds to wait") -> [_ _ _ _ _ _ _ _ _ _ _ _ _ _ _ _ _ _ _ _ _]
      tunnel: w356 -> [w369 _ _ _ _ _ _ _ _ _ _ _ _ _ _ _ _ _ _ _ _]
      tunnel: "Test Tree" -> [_ _ _ _ _ _ _ _ _ _ _ w584 w592 w594 w598 w606 _ _ _ _ _]
      tunnel: w355 -> [_ _ _ _ _ _ _ _ _ _ _ _ _ _ _ _ w619 _ w637 _ _]
      tunnel: w353 -> [_ _ _ _ _ _ _ _ _ _ _ _ _ _ _ _ w615 _ _ _ _]
      tunnel: w352 -> [_ _ _ _ _ _ _ _ _ _ _ _ _ _ _ _ w613 _ _ _ _]
      tunnel: w351 -> [w364 _ _ _ _ _ w535 _ _ _ _ _ _ _ _ _ _ _ _ _ _]
      tunnel: [w363 w412 w514 w519 w528 w532 w533 w542 w552 w559 w571 w583 w590 w593 w597 w605 w612 w632 w634 w638 w651] -> w350
      tunnel: w349 -> [w363 w412 w514 w519 w528 w532 w533 _ _ w559 w571 w583 w590 w593 w597 w605 w612 w632 w634 w638 w651]
      tunnel: w348 -> [w361 _ _ _ _ _ _ _ _ _ _ _ _ _ _ _ _ _ _ _ _]
      event Timeout {
        n209 = event-data() -> ()  [unwired: 1 in, 1 out]
        n210 = local read "Mode"() -> (w366:T4)
        n211 = case shown="\"Test\"" "Dashboard Tab" {
          tunnel: w369 -> [_ _ w385 _ _]
          tunnel: "TestMode/Automatic/" ("Name Pattern") -> [_ _ w384 _ _]
          tunnel: T20 [{"Operation"=enum."Clear", "Color Box"=14013909}, {"Operation"=enum."Clear", "Color Box"=14013909}, {"Operation"=enum."Clear", "Color Box"=14013909}, {"Operation"=enum."Clear", "Color Box"=14013909}, {"Operation"=enum."Update", "Color Box"=14013909}, {"Operation"=enum."Update", "Color Box"=16777215}, {"Operation"=enum."Clear", "Color Box"=14013909}, {"Operation"=enum."Clear", "Color Box"=14013909}, {"Operation"=enum."Clear", "Color Box"=14013909}] -> [_ _ w377 _ w405]
          tunnel: w366 -> [_ _ w376 _ w404]
          tunnel: u32[] [15790320, 15790320, 15790320, 15790320, 16777215, 16777215, 15790320, 15790320, 15790320] -> [_ _ _ _ w410]
          tunnel: w364 -> [_ _ _ _ w398]
          tunnel: w361 -> [_ w371 _ _ _]
          frame "Custom", Default {
          }
          frame "Basic" {
            n212 = call <vilib>:"WPI_DashboardUpdateNames.vi"("Controls on Tab"=w371) -> ()  [unwired: 11 in]
          }
          frame "Test" {
            w383 = -2 ("Active Item:Row Number")
            n213 = Index Array(array=w377, index=w376) -> (element=w378:T23)
            n214 = Unbundle(w378) -> ("Operation"=w379:enum16{"Update", "Clear"}, "Color Box"=w380:u32)
            n215 = call <vilib>:"NT Read String.vi"("Name"="TestMode/TestName") -> ("String"=w374:string)  [unwired: 9 in, 1 out]
            n216 = call <vilib>:"NT Read and Format Entries as Tree.vi"("Operation"=w379, "Name Pattern"=w384, "Tree Refnum"=w385) -> ()  [unwired: 7 in, 2 out]
            n217 = case shown="\"\"" w374 {
              tunnel: "TestMode/TestProgress" ("Name") -> [w387 _]
              tunnel: "TestMode/TestProgressText" ("Name") -> [w386 _]
              frame Default {
                n218 = call <vilib>:"NT Read Number.vi"("Name"=w387) -> ("Numeric"=w388:dbl)  [unwired: 9 in, 1 out]
                n219 = call <vilib>:"NT Read String.vi"("Name"=w386) -> ("String"=w389:string)  [unwired: 9 in, 1 out]
                n220 = Bundle("Numeric"=w388, "String"=w389) -> (→"Progress":cluster{"Numeric":dbl, "String":string})  [unwired: 1 in]
              }
              frame "" {
                n221 = property on="Progress" class="Clust (strict)"("Visible"=FALSE) -> ()  [unwired: 2 in, 2 out]
                n222 = local write "Test Name"(u16 0) -> ()
              }
            }
            n223 = property on="Test Tree" class="Tree (strict)"("Active Item Row Number"=w383, "ActiveColNum"=w383, "CellBG"=w380, "Active Item Row Number"=-1 ("Active Item:Row Number"), "CellBG"=u32 5789784 ("Color Box")) -> ()  [unwired: 2 in, 2 out]
          }
          frame "Variables" {
            w395 = string[] ["CameraPublisher", "Usage", "DB"]  # Items to initially close
            n224 = First Call?() -> (First Call?: T/F=w396:bool)
            n225 = control-ref of="Tree"() -> (w397:refnum<vi>)
            n226 = Select(t=w395, s=w396, f=string[] []) -> (s? t:f=w393:string[])
            n227 = call <vilib>:"NT Read and Format Entries as Tree.vi"("Tags to  Close"=w393, "Tree Refnum"=w397) -> ()  [unwired: 8 in, 2 out]
          }
          frame "Commands" {
            w406 = u32 5789784 ("Color Box")
            w407 = T24 {"Row"=-1, "Column"=-2} ("Active Cell:Active Cell")
            w409 = T24 {"Row"=-2, "Column"=-2} ("Active Cell:Active Cell")
            n228 = Index Array(array=w410, index=w404) -> (element=w408:u32)
            n229 = Index Array(array=w405, index=w404) -> (element=w403:T23)
            n230 = Unbundle(w403) -> ("Operation"=w402:enum16{"Update", "Clear"})  [unwired: 1 out]
            n231 = local read "Command Selection"() -> (w401:i32)
            n232 = property on="Command Selection" class="MCListbox (strict)"("ActiveCell"=w409, "CellBG"=w408, "ActiveCell"=w407, "CellBG"=w406) -> ()  [unwired: 2 in, 2 out]
            n233 = call <vilib>:"WPI_DashboardUpdate RPC Info.vi"("Operation"=w402) -> ("update"=w400:bool, "commands"=w399:string[][])  [unwired: 9 in]
            n234 = property on="Command Selection" class="MCListbox (strict)"("ItemNames"=w399) -> ()  [unwired: 2 in, 2 out]
            n235 = property on="Command Params" class="Tbl (strict)"("Active Cell"=w409, "Cell BG Color"=w408, "Active Cell"=w407, "Cell BG Color"=w406) -> ()  [unwired: 2 in, 2 out]
            n236 = call <vilib>:"WPI_DashboardUpdate Command Params.vi"("Update"=w400, "NewVal"=w401, "Commands"=w399, "Param Tbl"=w398) -> ()  [unwired: 7 in, 1 out]
          }
        }
        n237 = call <vilib>:"Connextion Info.vi"() -> ("Connected"=→"NT Connection":bool)  [unwired: 10 in, 1 out]
      }
      event "Test Tree": Value Change {
        # "Show appropriate\ncontrols"
        n238 = event-data() -> ("CtlRef"=w415:refnum<vi>, "NewVal"=w413:string)  [unwired: 1 in]
        n239 = call <vilib>:"WPI_UtilitiesGetTreeIOName.vi"("NewVal"=w413, "TreeControl in"=w415) -> ("I/O Name"=w416:string)  [unwired: 9 in]
        n240 = case shown="\"Camera\"" w416 {
          selector: w416 -> [_ w423 _ w445 w454 _]
          tunnel: w413 -> [_ _ w442 w444 _ w461]
          tunnel: cluster{string[]}[] [{["640x480", "320x240", "160x120"]}, {["Auto", "Fixed indoor", "Fixed outdoor 1", "Fixed outdoor 2", "Fixed fluorescent 1", "Fixed fluorescent 2", "Hold current"]}, {["Auto", "Flicker-free 50 Hz", "Flicker-free 60 Hz", "Hold current"]}, {["None", "Prioritize frame rate", "Prioritize image quality"]}, {["Monochrome", "Color"]}] -> [_ _ _ _ _ w460]
          frame Default {
            w418 = FALSE ("Visible")
            w417 = FALSE ("Visible")
            n241 = property on="Motor" class="Clust (strict)"("Visible"=w417) -> ()  [unwired: 2 in, 2 out]
            n242 = property on="Test Ring" class="Ring (strict)"("Visible"=w417) -> ()  [unwired: 2 in, 2 out]
            n243 = property on="Rev/Fwd" class="Clust (strict)"("Visible"=w418) -> ()  [unwired: 2 in, 2 out]
            n244 = property on="On/Off" class="Bool (strict)"("Visible"=w418) -> ()  [unwired: 2 in, 2 out]
            n245 = property on="Test Slider" class="Slide (strict)"("Visible"=w418) -> ()  [unwired: 2 in, 2 out]
          }
          frame "Analog Out", "Motor", "PWM" {
            w424 = FALSE ("Visible")
            n246 = case shown="\"Analog Out\"" w423 {
              tunnel: [1.0 ("Value") -1.0 ("Value") 0.0 ("Value")] -> w422
              tunnel: [255.0 ("Value") 1.0 ("Value") 5.0 ("Value")] -> w421
              tunnel: [128.0 ("Value") 0.0 ("Value") 0.0 ("Value")] -> w420
              tunnel: [64.0 ("Value") 0.5 ("Value") 1.0 ("Value")] -> w419
              frame "PWM" {
              }
              frame "Motor", Default {
              }
              frame "Analog Out" {
              }
            }
            n247 = property on="Motor" class="Clust (strict)"("Visible"=TRUE) -> ()  [unwired: 2 in, 2 out]
            n248 = property on="Value" class="Slide (strict)"("Value"=w420, "Scale.Minimum"=w422, "Scale.Maximum"=w421, "Scale.Increment"=w419) -> ()  [unwired: 2 in, 2 out]
            n249 = property on="On/Off" class="Bool (strict)"("Visible"=w424) -> ()  [unwired: 2 in, 2 out]
            n250 = property on="Test Slider" class="Slide (strict)"("Visible"=w424) -> ()  [unwired: 2 in, 2 out]
            n251 = property on="Test Ring" class="Ring (strict)"("Visible"=w424) -> ()  [unwired: 2 in, 2 out]
            n252 = property on="Rev/Fwd" class="Clust (strict)"("Visible"=w424) -> ()  [unwired: 2 in, 2 out]
          }
          frame "Servo" {
            w440 = FALSE ("Visible")
            n253 = call <vilib>:"NT Read Number.vi"("Name"=w442) -> ("Numeric"=w441:dbl)  [unwired: 9 in, 1 out]
            n254 = property on="Test Slider" class="Slide (strict)"("Visible"=TRUE, "Scale.Maximum"=170.0 ("Scale.Range:Maximum")) -> ()  [unwired: 2 in, 2 out]
            n255 = local write "Test Slider"(w441) -> ()
            n256 = property on="Motor" class="Clust (strict)"("Visible"=w440) -> ()  [unwired: 2 in, 2 out]
            n257 = property on="Rev/Fwd" class="Clust (strict)"("Visible"=w440) -> ()  [unwired: 2 in, 2 out]
            n258 = property on="On/Off" class="Bool (strict)"("Visible"=w440) -> ()  [unwired: 2 in, 2 out]
            n259 = property on="Test Ring" class="Ring (strict)"("Visible"=w440) -> ()  [unwired: 2 in, 2 out]
          }
          frame "Relay", "Solenoid" {
            w443 = FALSE ("Visible")
            n260 = property on="Motor" class="Clust (strict)"("Visible"=w443) -> ()  [unwired: 2 in, 2 out]
            n261 = property on="Test Slider" class="Slide (strict)"("Visible"=w443) -> ()  [unwired: 2 in, 2 out]
            n262 = Search and Replace String(input string=w444, search string="/Value  **", replace string="/Direction") -> (result string=w450:string)  [unwired: 5 in, 3 out]
            n263 = property on="Test Ring" class="Ring (strict)"("Visible"=w443) -> ()  [unwired: 2 in, 2 out]
            n264 = call <vilib>:"NT Read String.vi"("Name"=w450) -> ("String"=w448:string)  [unwired: 9 in, 1 out]
            n265 = Equal?(x="Both directions", y=w448) -> (x = y?=w446:bool)
            n266 = Not(x=w446) -> (.not. x?=w447:bool)
            n267 = property on="Rev/Fwd" class="Clust (strict)"("Visible"=w446) -> ()  [unwired: 2 in, 2 out]
            n268 = property on="On/Off" class="Bool (strict)"("Visible"=w447, "Caption.Text"=w445) -> ()  [unwired: 2 in, 2 out]
          }
          frame "Compressor", "Digital Out" {
            w453 = FALSE ("Visible")
            # "Get direction and finish"
            n269 = property on="Motor" class="Clust (strict)"("Visible"=w453) -> ()  [unwired: 2 in, 2 out]
            n270 = property on="Test Slider" class="Slide (strict)"("Visible"=w453) -> ()  [unwired: 2 in, 2 out]
            n271 = property on="Test Ring" class="Ring (strict)"("Visible"=w453) -> ()  [unwired: 2 in, 2 out]
            n272 = property on="On/Off" class="Bool (strict)"("Visible"=TRUE, "Caption.Text"=w454) -> ()  [unwired: 2 in, 2 out]
            n273 = property on="Rev/Fwd" class="Clust (strict)"("Visible"=FALSE) -> ()  [unwired: 2 in, 2 out]
          }
          frame "Camera" {
            n274 = call <vilib>:"Get Last Path Segment.vi"("String in"=w461) -> ("String out"=w462:string)  [unwired: 10 in]
            n275 = property on="On/Off" class="Bool (strict)"("Visible"=FALSE) -> ()  [unwired: 2 in, 2 out]
            n276 = property on="Motor" class="Clust (strict)"("Visible"=FALSE) -> ()  [unwired: 2 in, 2 out]
            n277 = property on="Rev/Fwd" class="Clust (strict)"("Visible"=FALSE) -> ()  [unwired: 2 in, 2 out]
            n278 = case shown="\"White Balance  **\"" w462 {
              tunnel: w461 -> [w468 w477 w486 w495 w504 _ w510]
              tunnel: w460 -> [w466 w474 w483 w492 w501 _ _]
              frame "Size  **" {
                n279 = Index Array(array=w466) -> (element=w465:cluster{string[]})  [unwired: 1 in]
                n280 = call <vilib>:"NT Read String.vi"("Name"=w468) -> ("String"=w467:string)  [unwired: 9 in, 1 out]
                n281 = Unbundle(w465) -> (w463:string[])
                n282 = Match First String(2:w463, 3:w467) -> (0:w464:i32)  [unwired: 1 out]
                n283 = property on="Test Ring" class="Ring (strict)"("Value"=w464, "Strings []"=w463) -> ()  [unwired: 2 in, 2 out]
                n284 = property on="Test Ring" class="Ring (strict)"("Visible"=TRUE) -> ()  [unwired: 2 in, 2 out]
                n285 = property on="Test Slider" class="Slide (strict)"("Visible"=FALSE) -> ()  [unwired: 2 in, 2 out]
              }
              frame "White Balance  **" {
                n286 = Index Array(array=w474, index=1) -> (element=w475:cluster{string[]})
                n287 = call <vilib>:"NT Read String.vi"("Name"=w477) -> ("String"=w476:string)  [unwired: 9 in, 1 out]
                n288 = Unbundle(w475) -> (w472:string[])
                n289 = Match First String(2:w472, 3:w476) -> (0:w471:i32)  [unwired: 1 out]
                n290 = property on="Test Ring" class="Ring (strict)"("Value"=w471, "Strings []"=w472) -> ()  [unwired: 2 in, 2 out]
                n291 = property on="Test Ring" class="Ring (strict)"("Visible"=TRUE) -> ()  [unwired: 2 in, 2 out]
                n292 = property on="Test Slider" class="Slide (strict)"("Visible"=FALSE) -> ()  [unwired: 2 in, 2 out]
              }
              frame "Exposure  **" {
                n293 = Index Array(array=w483, index=2) -> (element=w484:cluster{string[]})
                n294 = call <vilib>:"NT Read String.vi"("Name"=w486) -> ("String"=w485:string)  [unwired: 9 in, 1 out]
                n295 = Unbundle(w484) -> (w480:string[])
                n296 = Match First String(2:w480, 3:w485) -> (0:w481:i32)  [unwired: 1 out]
                n297 = property on="Test Ring" class="Ring (strict)"("Value"=w481, "Strings []"=w480) -> ()  [unwired: 2 in, 2 out]
                n298 = property on="Test Ring" class="Ring (strict)"("Visible"=TRUE) -> ()  [unwired: 2 in, 2 out]
                n299 = property on="Test Slider" class="Slide (strict)"("Visible"=FALSE) -> ()  [unwired: 2 in, 2 out]
              }
              frame "Exposure Priority  **" {
                n300 = Index Array(array=w492, index=3) -> (element=w493:cluster{string[]})
                n301 = call <vilib>:"NT Read String.vi"("Name"=w495) -> ("String"=w494:string)  [unwired: 9 in, 1 out]
                n302 = Unbundle(w493) -> (w489:string[])
                n303 = Match First String(2:w489, 3:w494) -> (0:w490:i32)  [unwired: 1 out]
                n304 = property on="Test Ring" class="Ring (strict)"("Value"=w490, "Strings []"=w489) -> ()  [unwired: 2 in, 2 out]
                n305 = property on="Test Ring" class="Ring (strict)"("Visible"=TRUE) -> ()  [unwired: 2 in, 2 out]
                n306 = property on="Test Slider" class="Slide (strict)"("Visible"=FALSE) -> ()  [unwired: 2 in, 2 out]
              }
              frame "Color Enable  **" {
                n307 = Index Array(array=w501, index=4) -> (element=w502:cluster{string[]})
                n308 = call <vilib>:"NT Read String.vi"("Name"=w504) -> ("String"=w503:string)  [unwired: 9 in, 1 out]
                n309 = Unbundle(w502) -> (w498:string[])
                n310 = Match First String(2:w498, 3:w503) -> (0:w499:i32)  [unwired: 1 out]
                n311 = property on="Test Ring" class="Ring (strict)"("Value"=w499, "Strings []"=w498) -> ()  [unwired: 2 in, 2 out]
                n312 = property on="Test Ring" class="Ring (strict)"("Visible"=TRUE) -> ()  [unwired: 2 in, 2 out]
                n313 = property on="Test Slider" class="Slide (strict)"("Visible"=FALSE) -> ()  [unwired: 2 in, 2 out]
              }
              frame Default {
                n314 = property on="Test Ring" class="Ring (strict)"("Visible"=FALSE) -> ()  [unwired: 2 in, 2 out]
                n315 = property on="Test Slider" class="Slide (strict)"("Visible"=FALSE) -> ()  [unwired: 2 in, 2 out]
              }
              frame "Brightness  **", "Color Level  **", "Compression  **", "FPS  **", "Sharpness  **" {
                n316 = call <vilib>:"NT Read Number.vi"("Name"=w510) -> ("Numeric"=w509:dbl)  [unwired: 9 in, 1 out]
                n317 = local write "Test Slider"(w509) -> ()
                n318 = property on="Test Slider" class="Slide (strict)"("Visible"=TRUE, "Scale.Maximum"=100.0 ("Scale.Range:Maximum")) -> ()  [unwired: 2 in, 2 out]
                n319 = property on="Test Ring" class="Ring (strict)"("Visible"=FALSE) -> ()  [unwired: 2 in, 2 out]
              }
            }
          }
        }
        n320 = property on="Progress" class="Clust (strict)"("Visible"=FALSE) -> ()  [unwired: 2 in, 2 out]
      }
      event "Test Name": Mouse Enter {
        # "Populate the ring with the list of tests"
        n321 = event-data() -> ()  [unwired: 1 in, 1 out]
        n322 = call <vilib>:"NT Read String Array.vi"("Name"="TestMode/TestList") -> ("String Array"=w518:string[])  [unwired: 9 in, 1 out]
        n323 = Build Array (concatenate)("Select the test to run...", w518) -> (w517:string[])
        n324 = property on="Test Name" class="Ring (strict)"("Strings []"=w517) -> ()  [unwired: 2 in, 2 out]
      }
      event "Test Name": Value Change {
        w520 = FALSE ("Visible")
        # "Tell the robot the test name to run"
        n325 = event-data() -> ("NewVal"=w524:u16)  [unwired: 1 in]
        n326 = property on="Test Name" class="Ring (strict)"() -> ("Strings []"=w525:string[])  [unwired: 2 in, 2 out]
        n327 = local write "Progress"(T6 {"Test Progress"=0, "Test Progress Text"=""} ("Progress")) -> ()
        n328 = Index Array(array=w525, index=w524) -> (element=w523:string)
        n329 = call <vilib>:"NT Write String.vi"("String"=w523, "Name"="TestMode/TestName") -> ()  [unwired: 9 in, 1 out]
        n330 = property on="Progress" class="Clust (strict)"("Visible"=TRUE) -> ()  [unwired: 2 in, 2 out]
        n331 = property on="Motor" class="Clust (strict)"("Visible"=w520) -> ()  [unwired: 2 in, 2 out]
        n332 = property on="Test Slider" class="Slide (strict)"("Visible"=w520) -> ()  [unwired: 2 in, 2 out]
        n333 = property on="On/Off" class="Bool (strict)"("Visible"=w520) -> ()  [unwired: 2 in, 2 out]
        n334 = property on="Rev/Fwd" class="Clust (strict)"("Visible"=w520) -> ()  [unwired: 2 in, 2 out]
        n335 = property on="Test Ring" class="Ring (strict)"("Visible"=w520) -> ()  [unwired: 2 in, 2 out]
      }
      event "Select Auto": Mouse Enter {
        # "Populate the combo box with the list of autonomous options"
        n336 = event-data() -> ()  [unwired: 1 in, 1 out]
        n337 = call <vilib>:"NT Read String Array.vi"("Name"="Auto List") -> ("String Array"=w527:string[])  [unwired: 9 in, 1 out]
        n338 = property on="Select Auto" class="CmbBox"("Strings[]"=w527) -> ()  [unwired: 2 in, 2 out]
      }
      event "Select Auto": Value Change {
        # "User modified the Auto Selection. Write to NT variable so robot knows."
        n339 = event-data() -> ("NewVal"=w530:string)  [unwired: 1 in]
        n340 = call <vilib>:"NT Write String.vi"("String"=w530, "Name"="Auto Selector") -> ()  [unwired: 9 in, 1 out]
      }
      event "Command Selection": Value Change {
        # "Get the params and show in table"
        n341 = event-data() -> ("NewVal"=w536:i32)  [unwired: 1 in]
        n342 = property on="Command Selection" class="MCListbox (strict)"() -> ("ItemNames"=w534:string[][])  [unwired: 2 in, 2 out]
        n343 = call <vilib>:"WPI_DashboardUpdate Command Params.vi"("NewVal"=w536, "Commands"=w534, "Param Tbl"=w535) -> ()  [unwired: 8 in, 1 out]
      }
      event "Execute Command": Value Change {
        # "Started one, Unique ID holds\nresponse"
        n344 = event-data() -> ()  [unwired: 1 in, 1 out]
        n345 = property on="Command Selection" class="MCListbox (strict)"() -> ("ItemNames"=w547:string[][])  [unwired: 2 in, 2 out]
        n346 = Index Array(array=w547, index (row)="Command Selection", index (col)=0) -> (element=w545:string)
        n347 = call <vilib>:"Invoke Commands.vi"("Command Params"="Command Params", "Function Name"=w545) -> ("Params"=w541:u8, "Started"=w540:bool)  [unwired: 7 in, 1 out]
        n348 = Array Subset(array="Command Params", length (row)=w541) -> (w542:string[][])  [unwired: 3 in]
        n349 = Select(t="Executing" ("Cmd Status"), s=w540, f="" ("Cmd Status")) -> (s? t:f=→"Cmd Status":string)
      }
      event "Command Selection": Double Click {
        n350 = event-data() -> ("Row"=w555:i32)  [unwired: 1 in]
        n351 = property on="Command Selection" class="MCListbox (strict)"() -> ("ItemNames"=w558:string[][])  [unwired: 2 in, 2 out]
        n352 = local read "Command Params"() -> (w554:string[][])
        n353 = Index Array(array=w558, index (row)=w555, index (col)=0) -> (element=w556:string)
        n354 = call <vilib>:"Invoke Commands.vi"("Command Params"=w554, "Function Name"=w556) -> ("Params"=w553:u8, "Started"=w548:bool)  [unwired: 7 in, 1 out]
        n355 = Array Subset(array=w554, length (row)=w553) -> (w552:string[][])  [unwired: 3 in]
        n356 = Select(t="Executing" ("Cmd Status"), s=w548, f="" ("Cmd Status")) -> (s? t:f=w549:string)
        n357 = local write "Cmd Status"(w549) -> ()
      }
      event "CheckList": Double Click {
        # "Shift clears all"
        # "Update symbols on the listbox"
        n358 = event-data() -> ("PlatMods.Shift"=w560:bool, "Row"=w562:i32)  [unwired: 1 in]
        n359 = case shown="True" w560 {
          tunnel: w562 -> [w566 _]
          tunnel: 1 -> [w565 _]
          frame False {
            n360 = property on="CheckList" class="LstBox (strict)"() -> ("Item Symbols"=w564:i32[])  [unwired: 2 in, 2 out]
            n361 = Replace Array Subset(array=w564, new element=w565, index=w566) -> (w563:i32[])
            n362 = property on="CheckList" class="LstBox (strict)"("Item Symbols"=w563) -> ()  [unwired: 2 in, 2 out]
          }
          frame True {
            w567 = 0 ("Top Row")
            n363 = property on="CheckList" class="LstBox (strict)"() -> ("Number of Rows"=w569:u32)  [unwired: 2 in, 2 out]
            n364 = Initialize Array(0, w569) -> (w568:i32[])
            n365 = property on="CheckList" class="LstBox (strict)"("Top Row"=w567, "Value"=w567, "Item Symbols"=w568) -> ()  [unwired: 2 in, 2 out]
          }
        }
      }
      event "CheckList": Key Down {
        # "Update symbols on the listbox\nLeft and right keys check and uncheck"
        n366 = event-data() -> ("VKey"=w573:T21)  [unwired: 1 in]
        n367 = case shown="\"Left\", \"Right\"" w573 {
          selector: w573 -> [w578 _]
          tunnel: eventvkey."Left" ("VKey") -> [w576 _]
          frame "Left", "Right" {
            n368 = Equal?(x=w576, y=w578) -> (x = y?=w577:bool)
            n369 = Select(t=0, s=w577, f=1) -> (s? t:f=w579:i32)
            n370 = property on="CheckList" class="LstBox (strict)"() -> ("Item Symbols"=w582:i32[])  [unwired: 2 in, 2 out]
            n371 = Replace Array Subset(array=w582, new element=w579, index="CheckList") -> (w581:i32[])
            n372 = property on="CheckList" class="LstBox (strict)"("Item Symbols"=w581) -> ()  [unwired: 2 in, 2 out]
          }
          frame Default {
          }
        }
      }
      event "Motor.Enable": Value Change {
        # "When the test mode otor enable helper is set, update that\ntree row item's value"
        n373 = event-data() -> ("NewVal"=w588:bool)  [unwired: 1 in]
        n374 = Unbundle("Motor") -> ("Value"=w587:dbl)  [unwired: 1 out]
        n375 = Select(t=w587, s=w588, f=0.0) -> (s? t:f=w585:dbl)
        n376 = call <vilib>:"NT Write Number.vi"("Numeric"=w585, "Name"=w584) -> ()  [unwired: 9 in, 1 out]
      }
      event "Test Slider": Value Change {
        # "When the test mode slider helper is set, update that\ntree row item's value"
        n377 = event-data() -> ("NewVal"=w591:dbl)  [unwired: 1 in]
        n378 = call <vilib>:"NT Write Number.vi"("Numeric"=w591, "Name"=w592) -> ()  [unwired: 9 in, 1 out]
      }
      event "On/Off": Value Change {
        # "When the test mode on/off helper value is set, update that\ntree row item's value"
        n379 = event-data() -> ("NewVal"=w596:bool)  [unwired: 1 in]
        n380 = Boolean To (0,1)(Boolean=w596) -> (0, 1=w595:i16)
        n381 = call <vilib>:"NT Write Number.vi"("Numeric"=w595, "Name"=w594) -> ()  [unwired: 9 in, 1 out]
      }
      event "Rev/Fwd": Value Change {
        # "When the test mode helper value for relays is set, update that\ntree row item's value"
        n382 = event-data() -> ("NewVal.Forward"=w604:bool, "NewVal.Reverse"=w603:bool)  [unwired: 1 in]
        n383 = Boolean To (0,1)(Boolean=w604) -> (0, 1=w600:i16)
        n384 = Boolean To (0,1)(Boolean=w603) -> (0, 1=w602:i16)
        n385 = Negate(x=w602) -> (-x=w601:i16)
        n386 = Add(x=w600, y=w601) -> (x+y=w599:i16)
        n387 = call <vilib>:"NT Write Number.vi"("Numeric"=w599, "Name"=w598) -> ()  [unwired: 9 in, 1 out]
      }
      event "Test Ring": Value Change {
        # "When a test mode helper value is selected from the ring,\nset the tree item's variable to the string value"
        n388 = event-data() -> ("NewVal"=w608:u16)  [unwired: 1 in]
        n389 = property on="Test Ring" class="Ring (strict)"() -> ("Strings []"=w609:string[])  [unwired: 2 in, 2 out]
        n390 = Index Array(array=w609, index=w608) -> (element=w607:string)
        n391 = call <vilib>:"NT Write String.vi"("String"=w607, "Name"=w606) -> ()  [unwired: 9 in, 1 out]
      }
      event "Rec Mode": Value Change {
        # "Update globals for recording mode and path to read log from.\nClear when logging and let NetworkTables set path for vision to\nuse."
        n392 = event-data() -> ("NewVal"=w620:enum32{"Stop", "Record", "Playback"})  [unwired: 1 in]
        n393 = global write "WPI_DashboardLogging Global.vi" "Logging Filename"(path "") -> ()
        n394 = global write "WPI_DashboardLogging Global.vi" "Recording"(w620) -> ()
        n395 = case shown="\"Playback\"" w620 {
          tunnel: w619 -> [_ w622 w631]
          tunnel: [_ _ w630] -> w617
          tunnel: [_ _ w629] -> _
          tunnel: w615 -> [_ _ w627]
          tunnel: cluster{i32, i32} {-250, 170} -> [_ _ w626]
          tunnel: [_ _ T22 {"Image Size"=TRUE, "Image Type"=TRUE, "Pixel Value"=TRUE, "ROI Information"=TRUE, "Zoom Factor"=FALSE} ("Image Information Shown:All Elements")] -> w610
          tunnel: [_ _ TRUE ("Zoom Factor")] -> w611
          tunnel: w613 -> [_ _ w623]
          frame Default {
          }
          frame "Stop", "Record" {
            # "Place Window too"
            n396 = invoke class="VI" method="FP.Close"(reference=w622) -> (reference out=w621:refnum<vi>)  [unwired: 2 in, 2 out]
            n397 = invoke class="VI" method="Abort VI"(reference=w621) -> ()  [unwired: 2 in, 3 out]
          }
          frame "Playback" {
            n398 = call "Open Playback Panel.vi"("Offset"=w626, "DB VI Ref"=w627, "Playback in"=w631) -> ("Playback out"=w628:refnum<vi>)  [unwired: 8 in]
            n399 = register-events(w628, w623) -> (reference out=w630:refnum<event-registration>, error out=w629:errorcluster)  [unwired: 2 in]
          }
        }
        n400 = property on="Camera Image Right" class="ImageControl"("Image Information Shown"=w610, "Image Information Visible"=w611) -> ()  [unwired: 2 in, 2 out]
        n401 = property on="Camera Image" class="ImageControl"("Image Information Shown"=w610, "Image Information Visible"=w611) -> ()  [unwired: 2 in, 2 out]
        n402 = call <vilib>:"WPI_DashboardNT Log FieldName Cache.vi"("Operation"=enum16{"Lookup/Add", "Index", "Clear"}."Clear") -> ()  [unwired: 8 in, 3 out]
      }
      event Panel Close {
        w633 = enum32{"Stop", "Record", "Playback"}."Stop" ("Rec Mode")
        # "Playback window has been closed, abort"
        n403 = event-data() -> ()  [unwired: 1 in, 4 out]
        n404 = local write "Rec Mode"(w633) -> ()
        n405 = global write "WPI_DashboardLogging Global.vi" "Recording"(w633) -> ()
      }
      event Panel Close {
        # "Abort playback window and ourself"
        n406 = event-data() -> ()  [unwired: 1 in, 4 out]
        n407 = invoke class="VI" method="FP.Close"(reference=w637) -> (reference out=w636:refnum<vi>)  [unwired: 2 in, 2 out]
        n408 = invoke class="VI" method="Abort VI"(reference=w636) -> (error out=w635:errorcluster)  [unwired: 2 in, 2 out]
        n409 = invoke class="VI" method="Abort VI"(error in=w635) -> ()  [unwired: 2 in, 3 out]
      }
      event User Event {
        n410 = event-data() -> ("IDs"=w644:cluster{"RPC field ID":u16, "Unique ID":u16}, "String"=w643:string)  [unwired: 1 in]
        n411 = Bundle("IDs"=w644, "String"=w643) -> (w642:T9)  [unwired: 1 in]
        n412 = call <vilib>:"Retrieve RPC Response.vi"("RPC Response"=w642) -> ("Output"=w640:string[][])  [unwired: 10 in]
        n413 = Build Array (concatenate)(w638, w640) -> (w639:string[][])
        n414 = local write "Command Params"(w639) -> ()
        n415 = local write "Cmd Status"("" ("Cmd Status")) -> ()
      }
      event "Tree": Double Click {
        n416 = event-data() -> ("PlatMods"=w650:T25, "Tag"=w647:string)  [unwired: 1 in]
        n417 = Unbundle(w650) -> ("Shift"=w649:bool)  [unwired: 4 out]
        n418 = String Subset(string=w647, length (rest)=1 ("length (rest)")) -> (substring=w646:string)  [unwired: 1 in]
        n419 = Not(x=w649) -> (.not. x?=w648:bool)
        n420 = case shown="\"/\"" w646 {
          tunnel: w647 -> [_ w653]
          tunnel: w648 -> [_ w652]
          frame Default {
          }
          frame "/" {
            n421 = call <vilib>:"NT Update Persistence.vi"("Persistence"=w652, "Name"=w653) -> ()  [unwired: 9 in, 1 out]
          }
        }
      }
    }
  }
  n422 = while {
    tunnel: w65 -> [w655]
    i -> [w658]
    stop <- FALSE stop-if-true
    n423 = Wait (ms)(milliseconds to wait=u32 100) -> ()  [unwired: 1 out]
    n424 = case shown="\"Playback\"" "Rec Mode" {
      tunnel: w658 -> [_ _ w673]
      tunnel: [u32 2829099 ("Base Color") u32 11141120 ("Target Color") w662] -> w654
      frame "Stop", Default {
        # "Reset the color, extra updates don't cost much"
      }
      frame "Record" {
      }
      frame "Playback" {
        # "Playback"
        n425 = Quotient & Remainder(x=w673, y=u32 50 ("milliseconds to wait")) -> (x-y*floor(x/y)=w669:u32)  [unwired: 1 out]
        n426 = Divide(x=w669, y=u32 50 ("milliseconds to wait")) -> (x/y=w666:dbl)
        n427 = Multiply(x=6.283185307179586, y=w666) -> (x*y=w671:dbl)
        n428 = Sine(x=w671) -> (sin(x)=w670:dbl)
        n429 = Absolute Value(x=w670) -> (abs(x)=w663:dbl)
        n430 = call "Interpolate RGB Color.vi"("Proportion"=w663, "Target Color"=u32 30976, "Base Color"=u32 2829099) -> ("Result Color"=w662:u32)  [unwired: 8 in]
      }
    }
    n431 = property class="Pane"(reference=w655, "PaneColor"=w654) -> ()  [unwired: 1 in, 2 out]
  }
  n432 = local write "Dashboard Tab"(T2."Drive" ("Dashboard Tab")) -> ()
  n433 = property on="On/Off" class="Bool (strict)"("Visible"=w36) -> ()  [unwired: 2 in, 2 out]
  n434 = property on="Motor" class="Clust (strict)"("Visible"=w36) -> ()  [unwired: 2 in, 2 out]
  n435 = property on="Progress" class="Clust (strict)"("Visible"=w36) -> ()  [unwired: 2 in, 2 out]
  n436 = property on="Test Ring" class="Ring (strict)"("Visible"=w36) -> ()  [unwired: 2 in, 2 out]
  n437 = property on="Rev/Fwd" class="Clust (strict)"("Visible"=w36) -> ()  [unwired: 2 in, 2 out]
  n438 = local write "Command Selection"(u16 0 ("milliseconds to wait")) -> ()
  n439 = while {
    tunnel: u16 1741 ("timeout ms (25000)") -> [w675]
    stop <- FALSE stop-if-true
    n440 = TCP Create Listener(10:w675) -> (0:w674:errorcluster, 3:w676:refnum<k5>)  [unwired: 4 in, 1 out]
    n441 = case shown="No Error" w674 {
      selector: w674 -> [w678 _]
      tunnel: w676 -> [w679 _]
      frame No Error {
        n442 = while {
          tunnel: w679 -> [w682]
          tunnel: w678 -> [w681]
          stop <- FALSE stop-if-true
          n443 = TCP Wait On Listener(8:w681, 11:w682) -> (0:w683:errorcluster, 4:w684:refnum<k5>)  [unwired: 2 in, 3 out]
          n444 = local write "TCP"(w684) -> ()
          n445 = case shown="No Error" w683 {
            frame No Error {
            }
            frame Error {
              n446 = Wait (ms)(milliseconds to wait=u32 1000) -> ()  [unwired: 1 out]
            }
          }
        }
      }
      frame Error {
        n447 = Wait (ms)(milliseconds to wait=u32 1000) -> ()  [unwired: 1 out]
      }
    }
  }
  n448 = local write "Command Params"(string[][] [] ("Command Params")) -> ()
  n449 = global write "WPI_DashboardLogging Global.vi" "Recording"(w59) -> ()
  n450 = local write "Rec Mode"(w59) -> ()
  n451 = call <vilib>:"NT Write String.vi"("String"="Select Auto", "Name"="Auto Selector") -> ()  [unwired: 9 in, 1 out]
